vi "combined.vi"() -> ()   [LabVIEW 2020]
uses:
  C:/Users/Public/Documents/Photometrics/PMQI-LabViewSamples/Examples/2018/Dependencies/PVCamNET.dll
  Dependencies/PVCamNET.dll
panel:
  out "SavingPath":string
  out "Boolean 2":bool
  in  "seq_close":bool
  out "Capturing":bool
  in  "seq_save":bool
  in  "seq_start":bool
  in  "Path":path
  in  "FramesToCapture":u16
  in  "Full CCD Height":u16
  in  "Full CCD Width":u16
  in  "Full CCD":bool
  in  "Get ROI":bool
  in  "Height":u16
  in  "Y":u16
  in  "Width":u16
  in  "X":u16
  out "Trigger Mode":i32
  in  "Trigger In Behaviour":string(combo)
  out "Exp. out":i32
  in  "Trigger Out Behaviour":string(combo)
  out "Boolean":bool
  in  "Scan Direction Reset":bool
  out "Scan Line Time":dbl format="%#_14g"
  in  "Scan Width":dbl
  in  "Scan Line Delay":dbl
  in  "Scan Direction":string(combo)
  in  "Scan Mode":string(combo)
  in  "Exposure Time":dbl
  in  "Live":bool
  in  "Camera Status":bool
  in  "Uninit":bool
  in  "Live stop":bool
  in  "Live start":bool
  in  "Open":bool
  # "Description:\nThis code lets the user use programmable scan\n mode for live imaging.\n\nSteps to run:\n1. Click \"Run\"\n2. Click \"Open\"\n3. Enter Exposure Time\n4. Select Scan Mode. \n5. Set Scan Line Delay or Scan Width\n6. Select Scan Direction\n7. Click \"Live start\"\n8. Click \"Live stop\"\n9. Right click on CamWindow and add a ROI.\n10. Click \"Get ROI\"\n11. Click \"Live start\"\n12. Click \"Live stop\"\n13. Right click on CamWindow and delete a ROI.\n14. Click \"Close\""
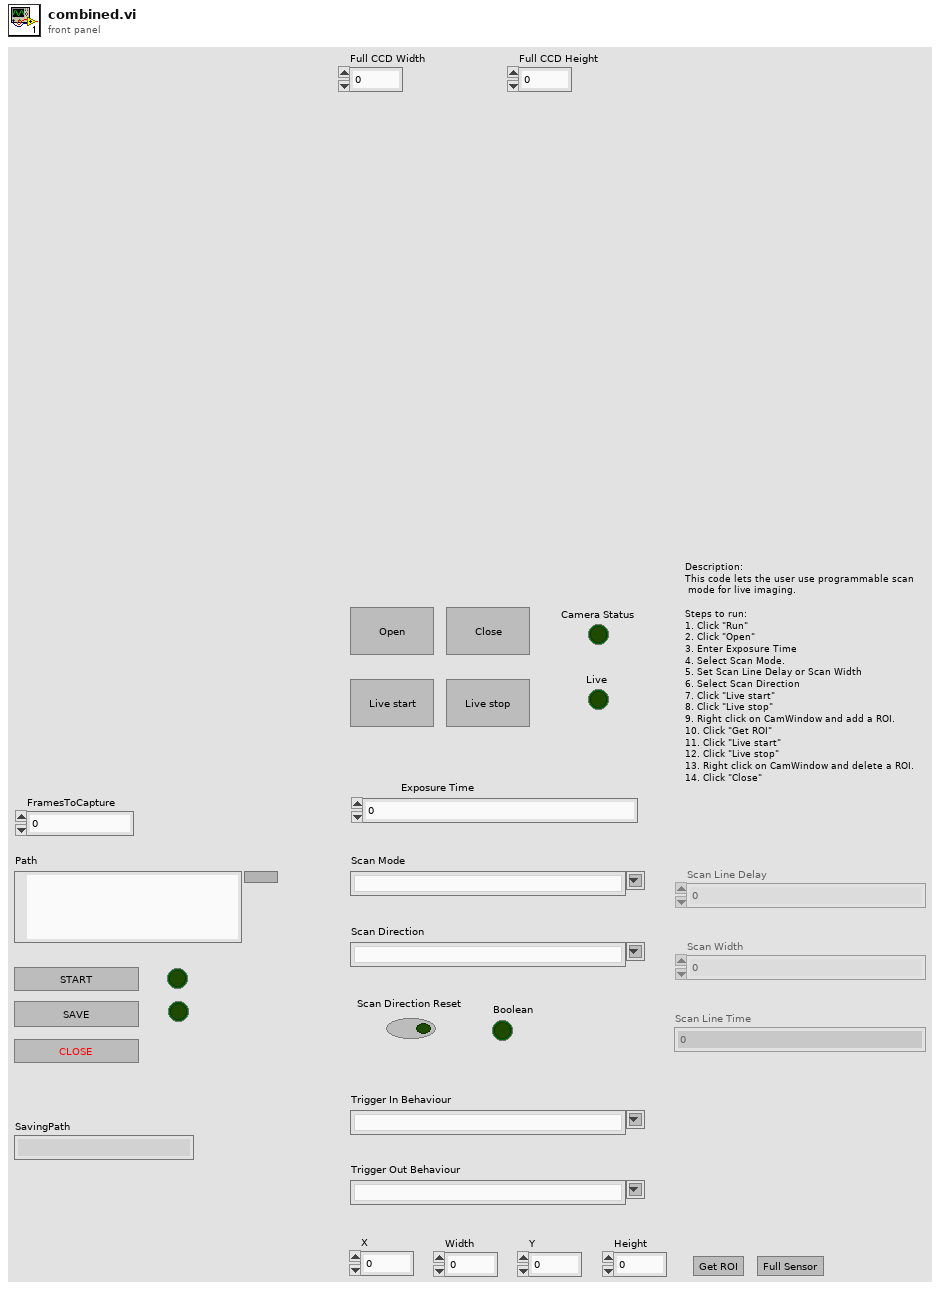
[diagram p1: front panel]
types:
  T1 = enum8{"Enabled", "Disabled", "Disabled and Grayed Out"}
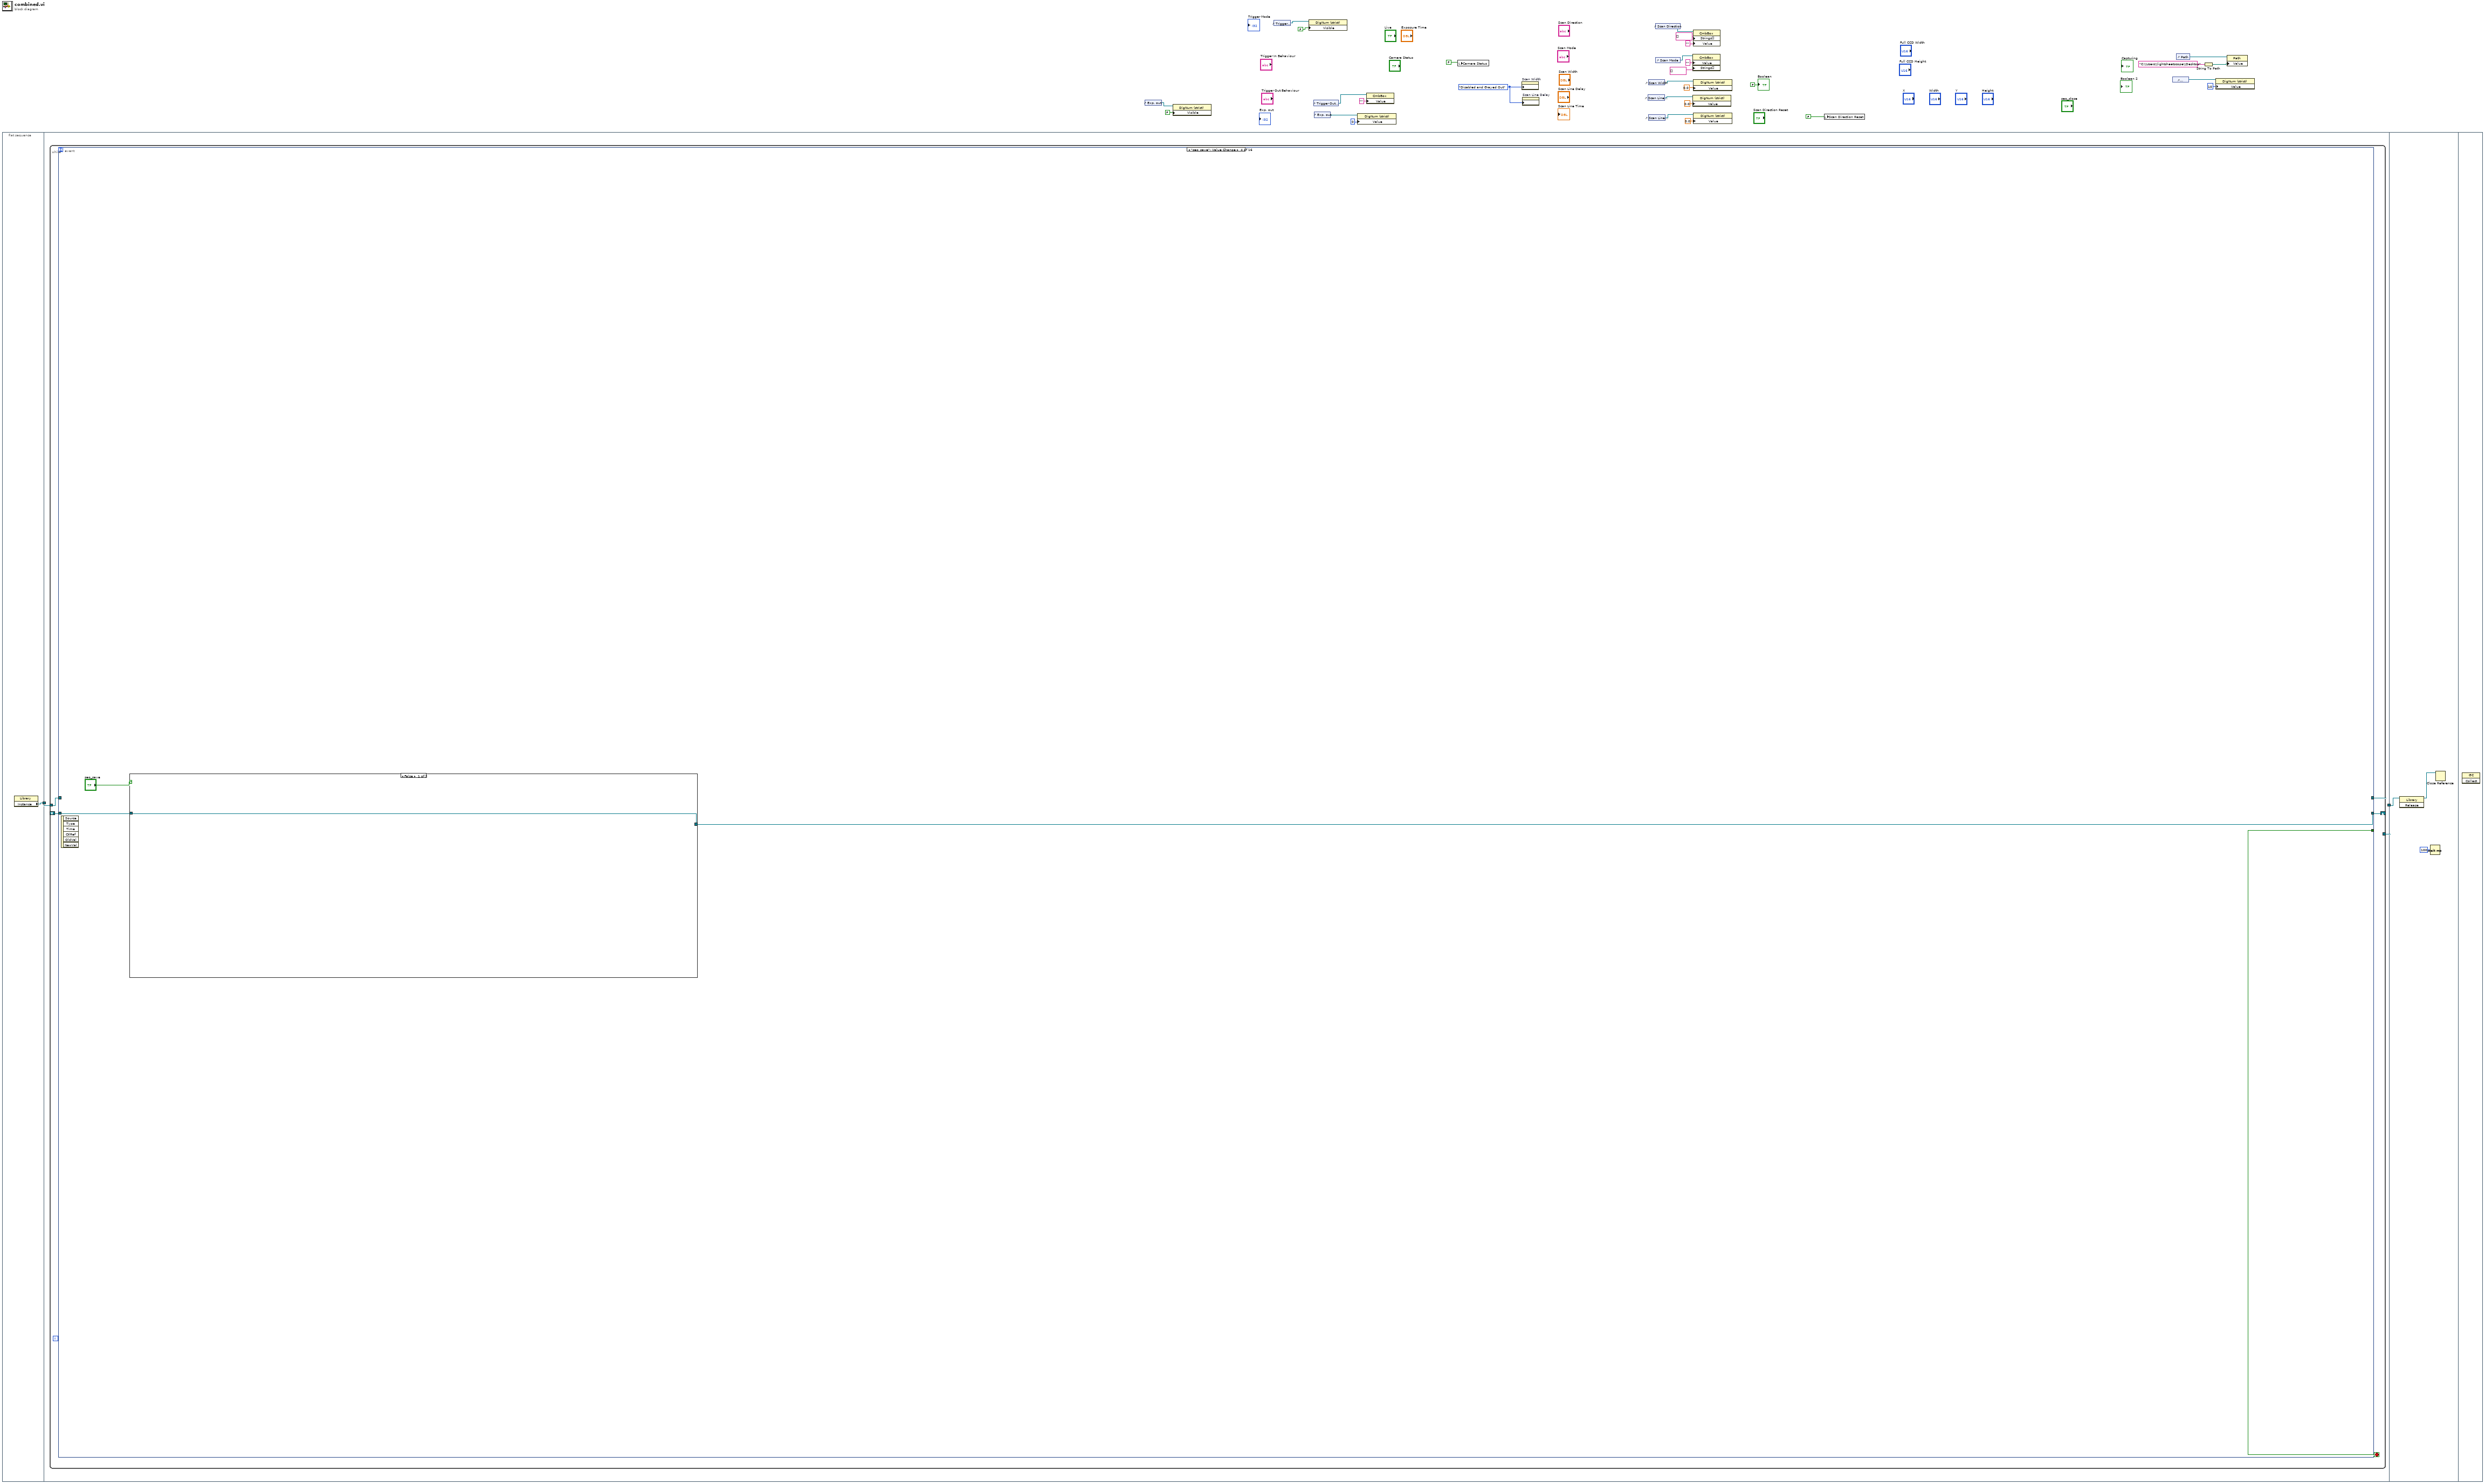
[diagram p0: block diagram]
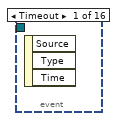
[diagram p2: hidden frame]
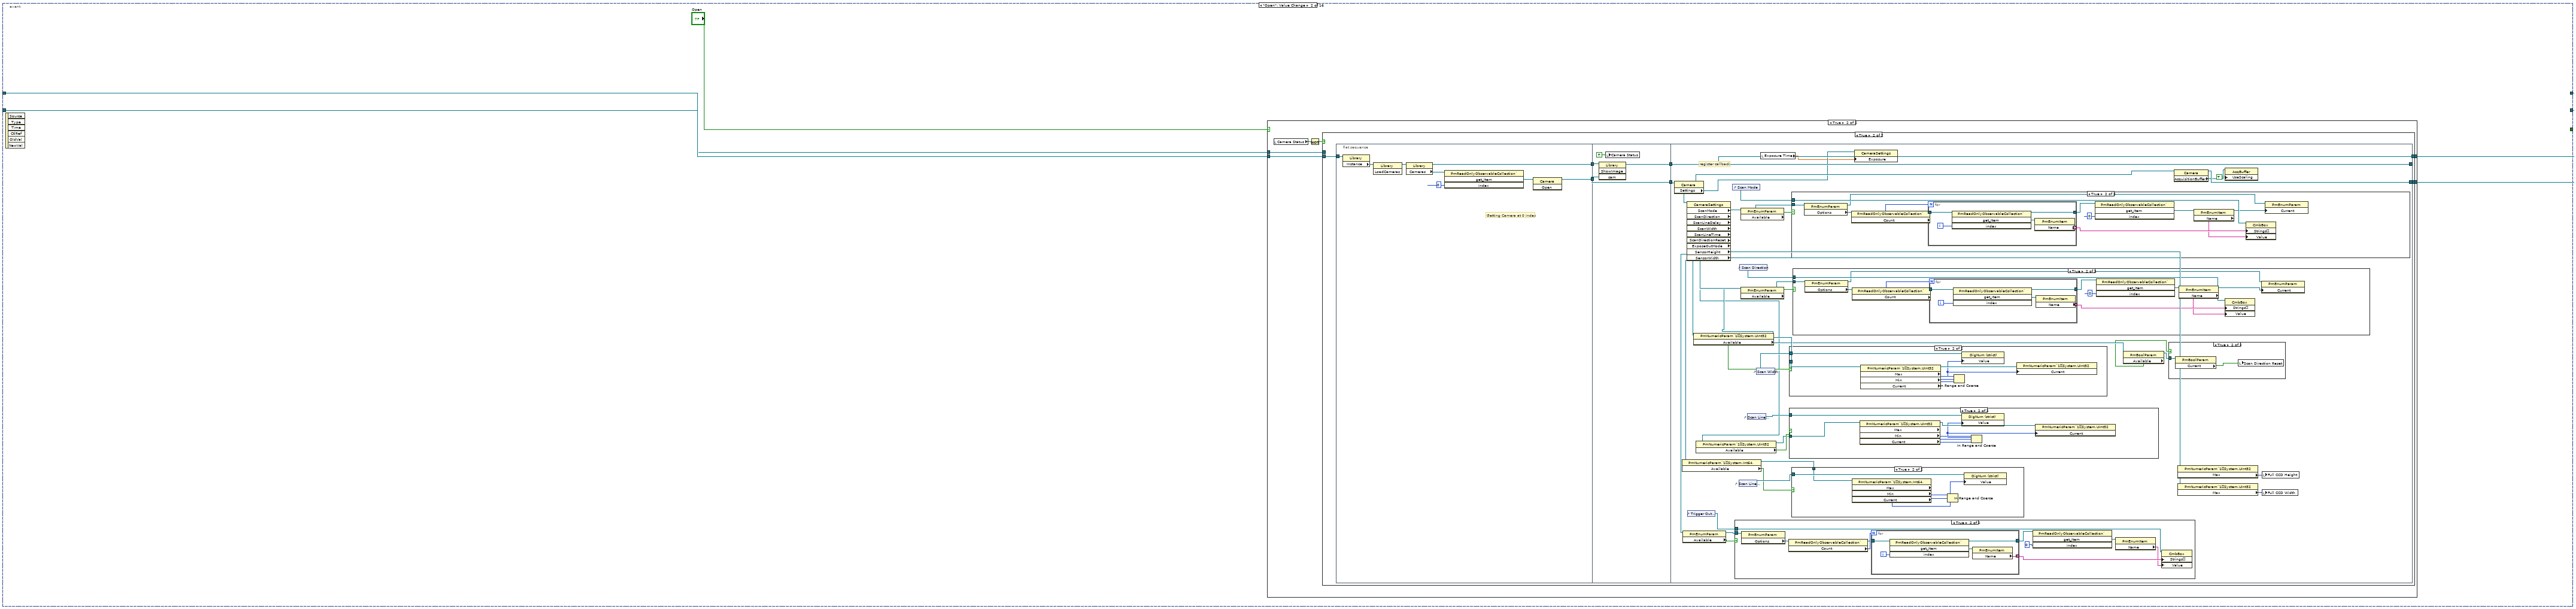
[diagram p3: hidden frame]
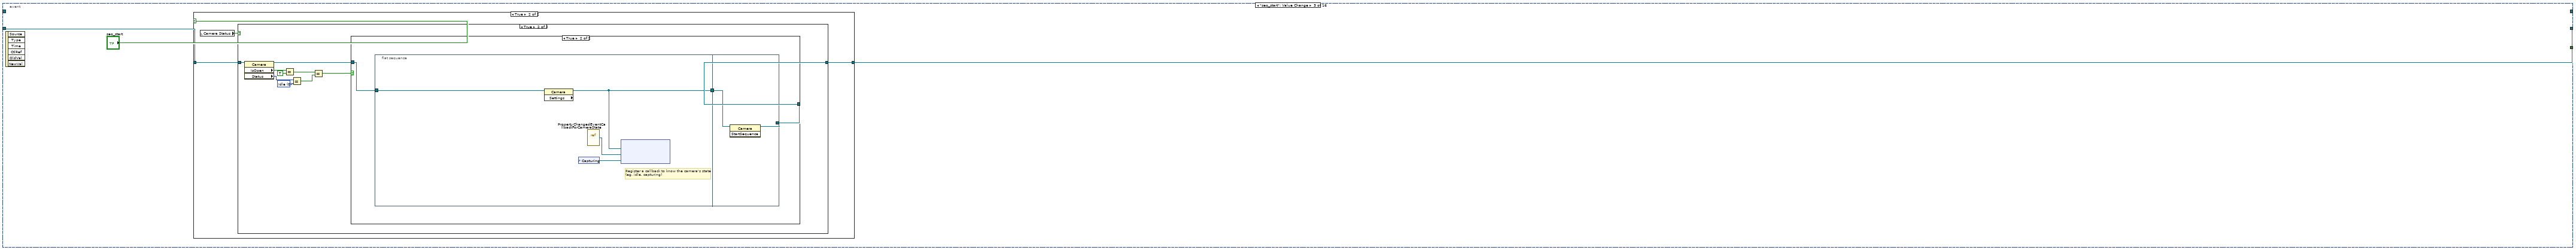
[diagram p13: hidden frame]
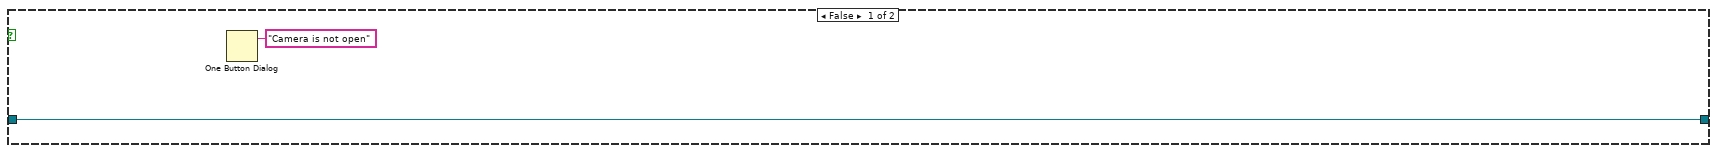
[diagram p15: hidden frame]
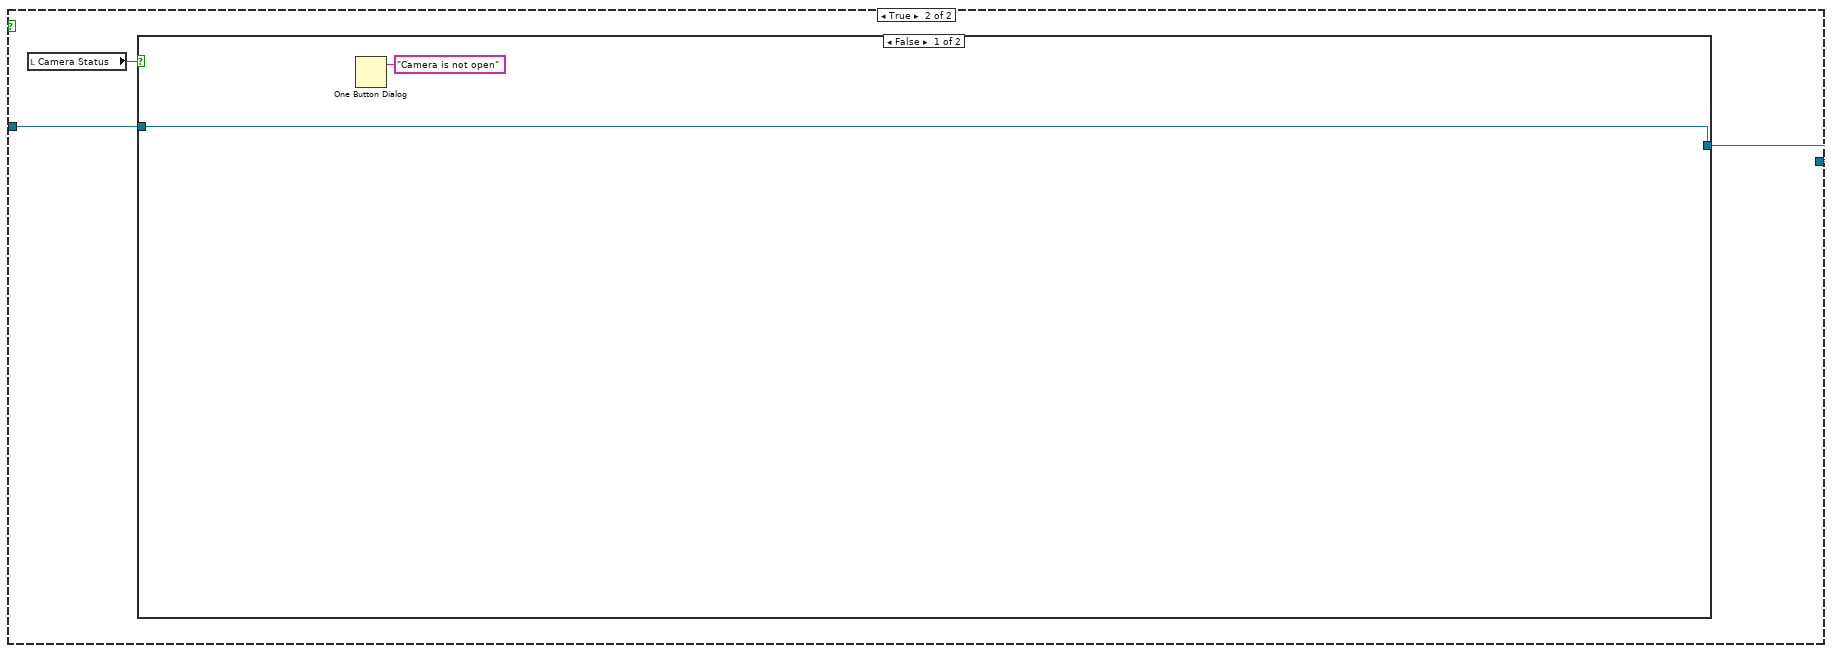
[diagram p17: hidden frame]
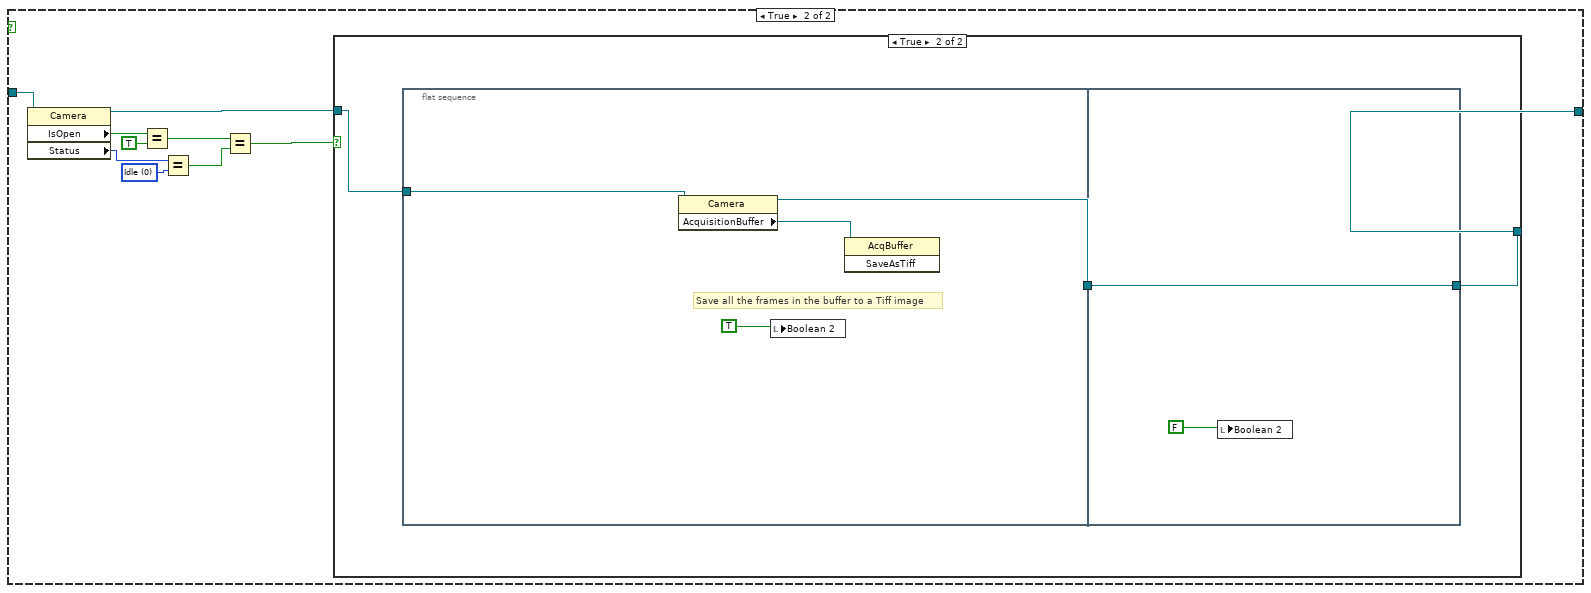
[diagram p18: hidden frame]
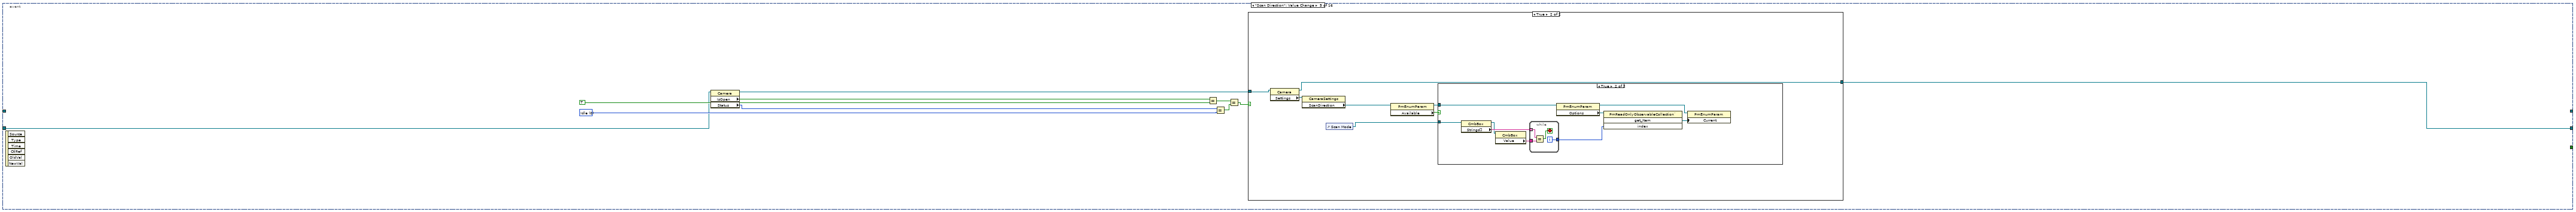
[diagram p20: hidden frame]
diagram:
  w16 = T1."Disabled and Grayed Out" ("Disabled")
  n1 = flat-sequence {
    tunnel: [w32] -> w31
    tunnel: w31 -> [w34]
    tunnel: [w33] -> w30
    tunnel: w30 -> [w855]
    frame #0 {
      n2 = property class="Library"() -> ("Instance"=w32:refnum<k24>)  [unwired: 2 in, 2 out]
    }
    frame #1 {
      n3 = while {
        tunnel: w34 -> [w39]
        shift-right: [w38] -> _
        shift-left: _ -> [w36]
        tunnel: [w37] -> w33
        stop <- w35 stop-if-true
        n4 = event shown="[3] \"seq_save\": Value Change" {
          selector: _ -> [_ _ _ _ _ _ _ _ _ _ _ _ _ _ _ _]
          dyn-events: _ -> [_ _ _ _ _ _ _ _ _ _ _ _ _ _ _ _]
          timeout: _ -> [_ _ _ _ _ _ _ _ _ _ _ _ _ _ _ _]
          tunnel: w39 -> [_ w44 _ _ _ _ _ _ w529 _ _ _ _ w772 _ w827]
          tunnel: [_ w43 w184 w215 w242 w274 w406 w470 w530 w597 w634 w707 w734 w773 w802 w828] -> w38
          tunnel: [_ w42 _ _ _ _ _ _ w529 _ _ _ _ w772 _ w827] -> w37
          tunnel: w36 -> [_ w41 w185 w214 w246 w275 w412 w472 w531 w598 w635 w708 w735 w774 w803 w829]
          tunnel: [_ _ _ _ _ _ _ _ _ _ _ _ _ _ _ w826] -> w35
          event Timeout {
            n5 = event-data() -> ()  [unwired: 1 in, 3 out]
          }
          event "Open": Value Change {
            n6 = event-data() -> ()  [unwired: 1 in, 6 out]
            n7 = case shown="True" "Open" {
              tunnel: w44 -> [w46 w52]
              tunnel: [w45 w51] -> w43
              tunnel: [w46 w50] -> w42
              tunnel: w41 -> [w45 w47]
              frame False {
              }
              frame True {
                n8 = local read "Camera Status"() -> (w49:bool)
                n9 = Not(x=w49) -> (.not. x?=w48:bool)
                n10 = case shown="True" w48 {
                  tunnel: w52 -> [w53 w59]
                  tunnel: [w54 w58] -> w51
                  tunnel: [w53 w57] -> w50
                  tunnel: w47 -> [w54 _]
                  frame False {
                  }
                  frame True {
                    n11 = flat-sequence {
                      tunnel: w59 -> [w64]
                      tunnel: [w66] -> w61
                      tunnel: [w65] -> w60
                      tunnel: w61 -> [w72]
                      tunnel: w60 -> [w73]
                      tunnel: [w73] -> w56
                      tunnel: [w71] -> w55
                      tunnel: [w112] -> w57
                      tunnel: [w92] -> w58
                      tunnel: w56 -> [w111]
                      tunnel: w55 -> [w112]
                      frame #0 {
                        # "Getting Camera at 0 index"
                        n12 = property class="Library"(reference=w64) -> ("Instance"=w63:refnum<k24>)  [unwired: 1 in, 2 out]
                        n13 = invoke class="Library" method="LoadCameras"(reference=w63) -> (reference out=w62:refnum<k24>)  [unwired: 2 in, 2 out]
                        n14 = property class="Library"(reference=w62) -> (reference out=w66:refnum<k24>, "Cameras"=w69:refnum<k24>)  [unwired: 1 in, 1 out]
                        n15 = invoke class="PmReadOnlyObservableCollection`" method="get_Item"(reference=w69, "index"=0) -> ("get_Item"=w67:refnum<k24>)  [unwired: 2 in, 3 out]
                        n16 = invoke class="Camera" method="Open"(reference=w67) -> (reference out=w65:refnum<k24>)  [unwired: 2 in, 2 out]
                      }
                      frame #1 {
                        n17 = invoke class="Library" method="ShowImage"(reference=w72, "cam"=w73) -> (reference out=w71:refnum<k24>)  [unwired: 2 in, 3 out]
                        n18 = local write "Camera Status"(TRUE ("Camera Status")) -> ()
                      }
                      frame #2 {
                        # "register callback"
                        n19 = property class="Camera"(reference=w111) -> (reference out=w93:refnum<k24>, "Settings"=w82:refnum<k24>)  [unwired: 1 in, 1 out]
                        n20 = property class="CameraSettings"(reference=w82) -> ("ScanMode"=w110:refnum<k24>, "ScanDirection"=w106:refnum<k24>, "ScanLineDelay"=w101:refnum<k24>, "ScanWidth"=w88:refnum<k24>, "ScanLineTime"=w80:refnum<k24>, "ScanDirectionReset"=w96:refnum<k24>, "ExposeOutMode"=w84:refnum<k24>, "SensorHeight"=w75:refnum<k24>, "SensorWidth"=w74:refnum<k24>)  [unwired: 1 in, 2 out]
                        n21 = property class="PmNumericParam`1[[System.Int64,"(reference=w80) -> (reference out=w78:refnum<k24>, "Available"=w79:bool)  [unwired: 1 in, 1 out]
                        n22 = property class="PmEnumParam"(reference=w84) -> (reference out=w85:refnum<k24>, "Available"=w86:bool)  [unwired: 1 in, 1 out]
                        n23 = control-ref of="Trigger Out Behaviour"() -> (w83:refnum<vi>)
                        n24 = property class="PmNumericParam`1[[System.UInt32"(reference=w101) -> (reference out=w99:refnum<k24>, "Available"=w100:bool)  [unwired: 1 in, 1 out]
                        n25 = property class="PmNumericParam`1[[System.UInt32"(reference=w88) -> (reference out=w87:refnum<k24>, "Available"=w89:bool)  [unwired: 1 in, 1 out]
                        n26 = control-ref of="Scan Mode"() -> (w107:refnum<vi>)
                        n27 = case shown="True" w86 {
                          tunnel: w85 -> [_ w122]
                          tunnel: w83 -> [_ w113]
                          frame False {
                          }
                          frame True {
                            n28 = property class="PmEnumParam"(reference=w122) -> ("Options"=w121:refnum<k24>)  [unwired: 1 in, 2 out]
                            n29 = property class="PmReadOnlyObservableCollection`"(reference=w121) -> (reference out=w119:refnum<k24>, "Count"=w120:i32)  [unwired: 1 in, 1 out]
                            n30 = for {
                              N: w120 -> [_]
                              tunnel: w119 -> [w127]
                              tunnel: [w124] -> w116
                              tunnel: [w123] -> w115 mode=indexing
                              i -> [w126]
                              n31 = invoke class="PmReadOnlyObservableCollection`" method="get_Item"(reference=w127, "index"=w126) -> (reference out=w124:refnum<k24>, "get_Item"=w125:refnum<k24>)  [unwired: 2 in, 2 out]
                              n32 = property class="PmEnumItem"(reference=w125) -> ("Name"=w123:string)  [unwired: 1 in, 2 out]
                            }
                            n33 = invoke class="PmReadOnlyObservableCollection`" method="get_Item"(reference=w116, "index"=0) -> ("get_Item"=w117:refnum<k24>)  [unwired: 2 in, 3 out]
                            n34 = property class="PmEnumItem"(reference=w117) -> ("Name"=w114:string)  [unwired: 1 in, 2 out]
                            n35 = property class="CmbBox"(reference=w113, "Strings[]"=w115, "Value"=w114) -> ()  [unwired: 1 in, 2 out]
                          }
                        }
                        n36 = control-ref of="Scan Line Time"() -> (w97:refnum<vi>)
                        n37 = control-ref of="Scan Direction"() -> (w103:refnum<vi>)
                        n38 = property class="PmEnumParam"(reference=w110) -> (reference out=w108:refnum<k24>, "Available"=w109:bool)  [unwired: 1 in, 1 out]
                        n39 = property class="PmEnumParam"(reference=w106) -> (reference out=w104:refnum<k24>, "Available"=w105:bool)  [unwired: 1 in, 1 out]
                        n40 = control-ref of="Scan Line Delay"() -> (w98:refnum<vi>)
                        n41 = control-ref of="Scan Width"() -> (w102:refnum<vi>)
                        n42 = local read "Exposure Time"() -> (w81:dbl)
                        n43 = case shown="True" w89 {
                          tunnel: w98 -> [_ w139]
                          tunnel: w87 -> [_ w138]
                          frame False {
                          }
                          frame True {
                            n44 = property class="PmNumericParam`1[[System.UInt32"(reference=w138) -> (reference out=w137:refnum<k24>, "Max"=w140:u32, "Min"=w141:u32, "Current"=w142:u32)  [unwired: 1 in, 1 out]
                            n45 = In Range and Coerce(upper limit=w140, x=w142, lower limit=w141) -> (coerced(x)=w136:u32)  [unwired: 1 out]
                            n46 = property class="DigNum (strict)"(reference=w139, "Value"=w136) -> ()  [unwired: 1 in, 2 out]
                            n47 = property class="PmNumericParam`1[[System.UInt32"(reference=w137, "Current"=w136) -> ()  [unwired: 1 in, 2 out]
                          }
                        }
                        n48 = case shown="True" w100 {
                          tunnel: w102 -> [_ w146]
                          tunnel: w99 -> [_ w145]
                          frame False {
                          }
                          frame True {
                            n49 = property class="PmNumericParam`1[[System.UInt32"(reference=w145) -> (reference out=w144:refnum<k24>, "Max"=w147:u32, "Min"=w148:u32, "Current"=w149:u32)  [unwired: 1 in, 1 out]
                            n50 = In Range and Coerce(upper limit=w147, x=w149, lower limit=w148) -> (coerced(x)=w143:u32)  [unwired: 1 out]
                            n51 = property class="DigNum (strict)"(reference=w146, "Value"=w143) -> ()  [unwired: 1 in, 2 out]
                            n52 = property class="PmNumericParam`1[[System.UInt32"(reference=w144, "Current"=w143) -> ()  [unwired: 1 in, 2 out]
                          }
                        }
                        n53 = case shown="True" w79 {
                          tunnel: w97 -> [_ w131]
                          tunnel: w78 -> [_ w130]
                          frame False {
                          }
                          frame True {
                            n54 = property class="PmNumericParam`1[[System.Int64,"(reference=w130) -> ("Max"=w132:i64, "Min"=w133:i64, "Current"=w134:i64)  [unwired: 1 in, 2 out]
                            n55 = In Range and Coerce(upper limit=w132, x=w134, lower limit=w133) -> (coerced(x)=w135:i64)  [unwired: 1 out]
                            n56 = property class="DigNum (strict)"(reference=w131, "Value"=w135) -> ()  [unwired: 1 in, 2 out]
                          }
                        }
                        n57 = case shown="True" w109 {
                          tunnel: w108 -> [_ w178]
                          tunnel: w107 -> [_ w170]
                          frame False {
                          }
                          frame True {
                            n58 = property class="PmEnumParam"(reference=w178) -> (reference out=w169:refnum<k24>, "Options"=w177:refnum<k24>)  [unwired: 1 in, 1 out]
                            n59 = property class="PmReadOnlyObservableCollection`"(reference=w177) -> (reference out=w175:refnum<k24>, "Count"=w176:i32)  [unwired: 1 in, 1 out]
                            n60 = for {
                              N: w176 -> [_]
                              tunnel: w175 -> [w183]
                              tunnel: [w180] -> w173
                              tunnel: [w179] -> w172 mode=indexing
                              i -> [w182]
                              n61 = invoke class="PmReadOnlyObservableCollection`" method="get_Item"(reference=w183, "index"=w182) -> (reference out=w180:refnum<k24>, "get_Item"=w181:refnum<k24>)  [unwired: 2 in, 2 out]
                              n62 = property class="PmEnumItem"(reference=w181) -> ("Name"=w179:string)  [unwired: 1 in, 2 out]
                            }
                            n63 = invoke class="PmReadOnlyObservableCollection`" method="get_Item"(reference=w173, "index"=0) -> ("get_Item"=w168:refnum<k24>)  [unwired: 2 in, 3 out]
                            n64 = property class="PmEnumItem"(reference=w168) -> (reference out=w167:refnum<k24>, "Name"=w171:string)  [unwired: 1 in, 1 out]
                            n65 = property class="CmbBox"(reference=w170, "Strings[]"=w172, "Value"=w171) -> ()  [unwired: 1 in, 2 out]
                            n66 = property class="PmEnumParam"(reference=w169, "Current"=w167) -> ()  [unwired: 1 in, 2 out]
                          }
                        }
                        n67 = case shown="True" w105 {
                          tunnel: w104 -> [_ w161]
                          tunnel: w103 -> [_ w152]
                          frame False {
                          }
                          frame True {
                            n68 = property class="PmEnumParam"(reference=w161) -> (reference out=w151:refnum<k24>, "Options"=w160:refnum<k24>)  [unwired: 1 in, 1 out]
                            n69 = property class="PmReadOnlyObservableCollection`"(reference=w160) -> (reference out=w158:refnum<k24>, "Count"=w159:i32)  [unwired: 1 in, 1 out]
                            n70 = for {
                              N: w159 -> [_]
                              tunnel: w158 -> [w166]
                              tunnel: [w163] -> w155
                              tunnel: [w162] -> w154 mode=indexing
                              i -> [w165]
                              n71 = invoke class="PmReadOnlyObservableCollection`" method="get_Item"(reference=w166, "index"=w165) -> (reference out=w163:refnum<k24>, "get_Item"=w164:refnum<k24>)  [unwired: 2 in, 2 out]
                              n72 = property class="PmEnumItem"(reference=w164) -> ("Name"=w162:string)  [unwired: 1 in, 2 out]
                            }
                            n73 = invoke class="PmReadOnlyObservableCollection`" method="get_Item"(reference=w155, "index"=0) -> ("get_Item"=w156:refnum<k24>)  [unwired: 2 in, 3 out]
                            n74 = property class="PmEnumItem"(reference=w156) -> (reference out=w150:refnum<k24>, "Name"=w153:string)  [unwired: 1 in, 1 out]
                            n75 = property class="CmbBox"(reference=w152, "Strings[]"=w154, "Value"=w153) -> ()  [unwired: 1 in, 2 out]
                            n76 = property class="PmEnumParam"(reference=w151, "Current"=w150) -> ()  [unwired: 1 in, 2 out]
                          }
                        }
                        n77 = property class="CameraSettings"(reference=w82, "Exposure"=w81) -> ()  [unwired: 1 in, 2 out]
                        n78 = property class="PmBoolParam"(reference=w96) -> (reference out=w94:refnum<k24>, "Available"=w95:bool)  [unwired: 1 in, 1 out]
                        n79 = case shown="True" w95 {
                          tunnel: w94 -> [_ w129]
                          frame False {
                          }
                          frame True {
                            n80 = property class="PmBoolParam"(reference=w129) -> ("Current"=w128:bool)  [unwired: 1 in, 2 out]
                            n81 = local write "Scan Direction Reset"(w128) -> ()
                          }
                        }
                        n82 = property class="Camera"(reference=w93) -> (reference out=w92:refnum<k24>, "AcquisitionBuffer"=w91:refnum<k24>)  [unwired: 1 in, 1 out]
                        n83 = property class="PmNumericParam`1[[System.UInt32"(reference=w75) -> ("Max"=w77:u32)  [unwired: 1 in, 2 out]
                        n84 = property class="PmNumericParam`1[[System.UInt32"(reference=w74) -> ("Max"=w76:u32)  [unwired: 1 in, 2 out]
                        n85 = property class="AcqBuffer"(reference=w91, "UseScaling"=TRUE) -> ()  [unwired: 1 in, 2 out]
                        n86 = local write "Full CCD Height"(w77) -> ()
                        n87 = local write "Full CCD Width"(w76) -> ()
                      }
                    }
                  }
                }
              }
            }
          }
          event "seq_start": Value Change {
            n88 = event-data() -> ()  [unwired: 1 in, 6 out]
            n89 = case shown="True" "seq_start" {
              tunnel: w185 -> [w187 w190]
              tunnel: [w187 w188] -> w184
              frame False {
              }
              frame True {
                n90 = local read "Camera Status"() -> (w189:bool)
                n91 = case shown="True" w189 {
                  tunnel: w190 -> [w191 w196]
                  tunnel: [w191 w193] -> w188
                  frame False {
                    n92 = One Button Dialog(message="Camera is not open") -> ()  [unwired: 1 in, 1 out]
                  }
                  frame True {
                    w201 = 0 items=["Idle", "Capturing"] ("Status")
                    n93 = property class="Camera"(reference=w196) -> (reference out=w195:refnum<k24>, "IsOpen"=w200:bool, "Status"=w202:i32)  [unwired: 1 in, 1 out]
                    n94 = Equal?(x=w200, y=TRUE) -> (x = y?=w198:bool)
                    n95 = Equal?(x=w202, y=w201) -> (x = y?=w197:bool)
                    n96 = Equal?(x=w198, y=w197) -> (x = y?=w194:bool)
                    n97 = case shown="True" w194 {
                      tunnel: w195 -> [w203 w206]
                      tunnel: [w203 w204] -> w193
                      frame False {
                      }
                      frame True {
                        n98 = flat-sequence {
                          tunnel: w206 -> [w208]
                          tunnel: [w207] -> w205
                          tunnel: [w212] -> w204
                          tunnel: w205 -> [w211]
                          frame #0 {
                            # "Register a callback to know the camera's state \n(eg. idle, capturing)"
                            n99 = property class="Camera" props=["Settings"](reference=w208) -> (reference out=w207:refnum<k24>)  [unwired: 1 in, 2 out]
                            n100 = control-ref of="Capturing"() -> (w209:refnum<vi>)
                            n101 = vi-ref "PropertyChangedEventCallbackForCameraState.vi"() -> ("vi reference"=w210:refnum<vi>)
                            n102 = node(w207, w210, w209) -> ()  [unwired: 2 in, 2 out]
                          }
                          frame #1 {
                            n103 = invoke class="Camera" method="StartSequence"(reference=w211) -> (reference out=w212:refnum<k24>)  [unwired: 2 in, 2 out]
                          }
                        }
                      }
                    }
                  }
                }
              }
            }
          }
          event "seq_save": Value Change {
            n104 = event-data() -> ()  [unwired: 1 in, 6 out]
            n105 = case shown="False" "seq_save" {
              tunnel: [w216 w218] -> w215
              tunnel: w214 -> [w216 w217]
              frame False {
              }
              frame True {
                n106 = local read "Camera Status"() -> (w219:bool)
                n107 = case shown="False" w219 {
                  tunnel: [w220 w223] -> w218
                  tunnel: w217 -> [w220 w222]
                  frame False {
                    n108 = One Button Dialog(message="Camera is not open") -> ()  [unwired: 1 in, 1 out]
                  }
                  frame True {
                    w230 = 0 items=["Idle", "Capturing"] ("Status")
                    n109 = property class="Camera"(reference=w222) -> (reference out=w225:refnum<k24>, "IsOpen"=w229:bool, "Status"=w231:i32)  [unwired: 1 in, 1 out]
                    n110 = Equal?(x=w229, y=TRUE) -> (x = y?=w227:bool)
                    n111 = Equal?(x=w231, y=w230) -> (x = y?=w226:bool)
                    n112 = Equal?(x=w227, y=w226) -> (x = y?=w224:bool)
                    n113 = case shown="True" w224 {
                      tunnel: w225 -> [w232 w235]
                      tunnel: [w232 w234] -> w223
                      frame False {
                      }
                      frame True {
                        n114 = flat-sequence {
                          tunnel: [w237] -> w233
                          tunnel: w235 -> [w236]
                          tunnel: [w240] -> w234
                          tunnel: w233 -> [w240]
                          frame #0 {
                            # "Save all the frames in the buffer to a Tiff image"
                            n115 = property class="Camera"(reference=w236) -> (reference out=w237:refnum<k24>, "AcquisitionBuffer"=w239:refnum<k24>)  [unwired: 1 in, 1 out]
                            n116 = local write "Boolean 2"(TRUE ("Camera Status")) -> ()
                            n117 = invoke class="AcqBuffer" method="SaveAsTiff"(reference=w239) -> ()  [unwired: 2 in, 3 out]
                          }
                          frame #1 {
                            n118 = local write "Boolean 2"(FALSE ("Camera Status")) -> ()
                          }
                        }
                      }
                    }
                  }
                }
              }
            }
          }
          event "Scan Direction": Value Change {
            w250 = 0 items=["Idle", "Capturing"] ("Status")
            n119 = event-data() -> ()  [unwired: 1 in, 6 out]
            n120 = property class="Camera"(reference=w246) -> (reference out=w243:refnum<k24>, "IsOpen"=w249:bool, "Status"=w251:i32)  [unwired: 1 in, 1 out]
            n121 = Equal?(x=w249, y=TRUE) -> (x = y?=w245:bool)
            n122 = Equal?(x=w251, y=w250) -> (x = y?=w247:bool)
            n123 = Equal?(x=w245, y=w247) -> (x = y?=w244:bool)
            n124 = case shown="True" w244 {
              tunnel: w243 -> [w252 w256]
              tunnel: [w252 w253] -> w242
              frame False {
              }
              frame True {
                n125 = property class="Camera"(reference=w256) -> (reference out=w253:refnum<k24>, "Settings"=w257:refnum<k24>)  [unwired: 1 in, 1 out]
                n126 = property class="CameraSettings"(reference=w257) -> ("ScanDirection"=w255:refnum<k24>)  [unwired: 1 in, 2 out]
                n127 = control-ref of="Scan Mode"() -> (w254:refnum<vi>)
                n128 = property class="PmEnumParam"(reference=w255) -> (reference out=w258:refnum<k24>, "Available"=w259:bool)  [unwired: 1 in, 1 out]
                n129 = case shown="True" w259 {
                  tunnel: w258 -> [_ w267]
                  tunnel: w254 -> [_ w260]
                  frame False {
                  }
                  frame True {
                    n130 = property class="CmbBox"(reference=w260) -> (reference out=w262:refnum<vi>, "Strings[]"=w268:string[])  [unwired: 1 in, 1 out]
                    n131 = property class="CmbBox"(reference=w262) -> ("Value"=w261:string)  [unwired: 1 in, 2 out]
                    n132 = while {
                      tunnel: w268 -> [w272] mode=indexing
                      tunnel: [w270] -> w265
                      tunnel: w261 -> [w269]
                      i -> [w270]
                      stop <- w271 stop-if-true
                      n133 = Equal?(x=w272, y=w269) -> (x = y?=w271:bool)
                    }
                    n134 = property class="PmEnumParam"(reference=w267) -> (reference out=w264:refnum<k24>, "Options"=w266:refnum<k24>)  [unwired: 1 in, 1 out]
                    n135 = invoke class="PmReadOnlyObservableCollection`" method="get_Item"(reference=w266, "index"=w265) -> ("get_Item"=w263:refnum<k24>)  [unwired: 2 in, 3 out]
                    n136 = property class="PmEnumParam"(reference=w264, "Current"=w263) -> ()  [unwired: 1 in, 2 out]
                  }
                }
              }
            }
          }
          event "Scan Mode", "Scan Direction Reset": Value Change {
            n137 = event-data() -> ()  [unwired: 1 in, 6 out]
            n138 = local read "Camera Status"() -> (w273:bool)
            n139 = case shown="True" w273 {
              tunnel: w275 -> [w276 w281]
              tunnel: [w276 w279] -> w274
              frame False {
                n140 = One Button Dialog(message="Camera is not open") -> ()  [unwired: 1 in, 1 out]
              }
              frame True {
                w286 = 0 items=["Idle", "Capturing"] ("Status")
                n141 = property class="Camera"(reference=w281) -> (reference out=w280:refnum<k24>, "IsOpen"=w285:bool, "Status"=w287:i32)  [unwired: 1 in, 1 out]
                n142 = Equal?(x=w285, y=TRUE) -> (x = y?=w283:bool)
                n143 = Equal?(x=w287, y=w286) -> (x = y?=w282:bool)
                n144 = Equal?(x=w283, y=w282) -> (x = y?=w278:bool)
                n145 = case shown="True" w278 {
                  tunnel: w280 -> [w288 w327]
                  tunnel: [w288 w322] -> w279
                  frame False {
                  }
                  frame True {
                    # "For Scan mode type if Auto is chosen then Scan Width and Scan Line Delay are not configurable.\nIf Line Delay is chosen then Scan Line is configurable, but Scan Width is not configurable.\nSimilarly if Scan Delay is chosen then Scan Line Delay is configurable, but Scan Width is not configurable."
                    n146 = property class="Camera"(reference=w327) -> (reference out=w322:refnum<k24>, "Settings"=w326:refnum<k24>)  [unwired: 1 in, 1 out]
                    n147 = property class="CameraSettings"(reference=w326) -> (error out=w319:errorcluster, "ScanMode"=w325:refnum<k24>, "ScanDirection"=w321:refnum<k24>, "ScanWidth"=w317:refnum<k24>, "ScanLineDelay"=w316:refnum<k24>, "ScanLineTime"=w305:refnum<k24>, "ScanDirectionReset"=w294:refnum<k24>)  [unwired: 1 in, 1 out]
                    n148 = control-ref of="Scan Line Delay"() -> (w296:refnum<vi>)
                    n149 = control-ref of="Scan Line Time"() -> (w299:refnum<vi>)
                    n150 = control-ref of="Scan Width"() -> (w312:refnum<vi>)
                    n151 = property class="PmEnumParam"(reference=w325, error in=w319) -> (reference out=w323:refnum<k24>, error out=w320:errorcluster, "Available"=w324:bool)
                    n152 = control-ref of="Scan Mode"() -> (w318:refnum<vi>)
                    n153 = control-ref of="Scan Direction"() -> (w315:refnum<vi>)
                    n154 = case shown="True" w324 {
                      tunnel: w323 -> [_ w400]
                      tunnel: w318 -> [_ w395]
                      tunnel: w320 -> [w388 w394]
                      tunnel: [w388 w389] -> w304
                      frame False {
                      }
                      frame True {
                        n155 = property class="CmbBox"(reference=w395) -> (reference out=w396:refnum<vi>, "Strings[]"=w401:string[])  [unwired: 1 in, 1 out]
                        n156 = property class="CmbBox"(reference=w396) -> ("Value"=w391:string)  [unwired: 1 in, 2 out]
                        n157 = while {
                          tunnel: w401 -> [w405] mode=indexing
                          tunnel: [w403] -> w398
                          tunnel: w391 -> [w402]
                          i -> [w403]
                          stop <- w404 stop-if-true
                          n158 = Equal?(x=w405, y=w402) -> (x = y?=w404:bool)
                        }
                        n159 = property class="PmEnumParam"(reference=w400, error in=w394) -> (reference out=w397:refnum<k24>, error out=w393:errorcluster, "Options"=w399:refnum<k24>)
                        n160 = invoke class="PmReadOnlyObservableCollection`" method="get_Item"(reference=w399, error in=w393, "index"=w398) -> (error out=w392:errorcluster, "get_Item"=w390:refnum<k24>)  [unwired: 1 in, 2 out]
                        n161 = property class="PmEnumParam" props=["Current", "IsReadOnly"](reference=w397, error in=w392, "Current"=w390) -> (error out=w389:errorcluster)  [unwired: 2 out]
                      }
                    }
                    n162 = property class="PmEnumParam"(reference=w321, error in=w304) -> (reference out=w313:refnum<k24>, error out=w307:errorcluster, "Available"=w314:bool)
                    n163 = case shown="True" w314 {
                      tunnel: w313 -> [_ w382]
                      tunnel: w315 -> [_ w374]
                      tunnel: w307 -> [w366 w373]
                      tunnel: [w366 w367] -> w306
                      frame False {
                      }
                      frame True {
                        n164 = property class="PmEnumParam"(reference=w382, error in=w373) -> (reference out=w368:refnum<k24>, error out=w372:errorcluster, "Options"=w381:refnum<k24>)
                        n165 = property class="PmReadOnlyObservableCollection`"(reference=w381) -> (reference out=w379:refnum<k24>, "Count"=w380:i32)  [unwired: 1 in, 1 out]
                        n166 = for {
                          N: w380 -> [_]
                          tunnel: w379 -> [w387]
                          tunnel: [w384] -> w377
                          tunnel: [w383] -> w376 mode=indexing
                          i -> [w386]
                          n167 = invoke class="PmReadOnlyObservableCollection`" method="get_Item"(reference=w387, "index"=w386) -> (reference out=w384:refnum<k24>, "get_Item"=w385:refnum<k24>)  [unwired: 2 in, 2 out]
                          n168 = property class="PmEnumItem"(reference=w385) -> ("Name"=w383:string)  [unwired: 1 in, 2 out]
                        }
                        n169 = invoke class="PmReadOnlyObservableCollection`" method="get_Item"(reference=w377, error in=w372, "index"=0) -> (error out=w371:errorcluster, "get_Item"=w369:refnum<k24>)  [unwired: 1 in, 2 out]
                        n170 = property class="PmEnumItem"(reference=w369, error in=w371) -> (error out=w370:errorcluster, "Name"=w375:string)  [unwired: 1 out]
                        n171 = property class="CmbBox"(reference=w374, error in=w370, "Strings[]"=w376, "Value"=w375) -> (error out=w367:errorcluster)  [unwired: 1 out]
                        n172 = property class="PmEnumParam"(reference=w368, "Current"=w369) -> ()  [unwired: 1 in, 2 out]
                      }
                    }
                    n173 = property class="PmNumericParam`1[[System.UInt32"(reference=w317, error in=w306) -> (reference out=w310:refnum<k24>, error out=w309:errorcluster, "Available"=w311:bool)
                    n174 = case shown="True" w311 {
                      tunnel: w312 -> [_ w362]
                      tunnel: w310 -> [_ w359]
                      tunnel: w309 -> [w356 w361]
                      tunnel: [w356 w360] -> w308
                      frame False {
                      }
                      frame True {
                        n175 = property class="PmNumericParam`1[[System.UInt32"(reference=w359) -> ("Current"=w363:u32, "IsReadOnly"=w358:bool)  [unwired: 1 in, 2 out]
                        n176 = case shown="False" w358 {
                          tunnel: [T1."Enabled" ("Disabled") T1."Disabled and Grayed Out" ("Disabled")] -> w357
                          frame False {
                          }
                          frame True {
                          }
                        }
                        n177 = property class="DigNum (strict)"(reference=w362, error in=w361, "Value"=w363, "DisabledEnum"=w357) -> (error out=w360:errorcluster)  [unwired: 1 out]
                      }
                    }
                    n178 = property class="PmNumericParam`1[[System.UInt32"(reference=w316, error in=w308) -> (reference out=w301:refnum<k24>, error out=w295:errorcluster, "Available"=w302:bool)
                    n179 = case shown="True" w302 {
                      tunnel: w296 -> [_ w352]
                      tunnel: w301 -> [_ w349]
                      tunnel: w295 -> [w346 w351]
                      tunnel: [w346 w350] -> w298
                      frame False {
                      }
                      frame True {
                        n180 = property class="PmNumericParam`1[[System.UInt32"(reference=w349) -> ("Current"=w353:u32, "IsReadOnly"=w348:bool)  [unwired: 1 in, 2 out]
                        n181 = case shown="False" w348 {
                          tunnel: [T1."Enabled" ("Disabled") T1."Disabled and Grayed Out" ("Disabled")] -> w347
                          frame False {
                          }
                          frame True {
                          }
                        }
                        n182 = property class="DigNum (strict)"(reference=w352, error in=w351, "Value"=w353, "DisabledEnum"=w347) -> (error out=w350:errorcluster)  [unwired: 1 out]
                      }
                    }
                    n183 = property class="PmNumericParam`1[[System.Int64,"(reference=w305, error in=w298) -> (reference out=w300:refnum<k24>, error out=w297:errorcluster, "Available"=w303:bool)
                    n184 = case shown="True" w303 {
                      tunnel: w299 -> [_ w342]
                      tunnel: w300 -> [_ w339]
                      tunnel: w297 -> [w336 w341]
                      tunnel: [w336 w340] -> w290
                      frame False {
                      }
                      frame True {
                        n185 = property class="PmNumericParam`1[[System.Int64,"(reference=w339) -> ("Current"=w343:i64, "IsReadOnly"=w338:bool)  [unwired: 1 in, 2 out]
                        n186 = case shown="False" w338 {
                          tunnel: [T1."Enabled" ("Disabled") T1."Disabled and Grayed Out" ("Disabled")] -> w337
                          frame False {
                          }
                          frame True {
                          }
                        }
                        n187 = property class="DigNum (strict)"(reference=w342, error in=w341, "Value"=w343, "DisabledEnum"=w337) -> (error out=w340:errorcluster)  [unwired: 1 out]
                      }
                    }
                    n188 = property class="PmBoolParam"(reference=w294, error in=w290) -> (reference out=w292:refnum<k24>, error out=w289:errorcluster, "Available"=w293:bool)
                    n189 = control-ref of="Scan Direction Reset"() -> (w291:refnum<vi>)
                    n190 = case shown="True" w293 {
                      tunnel: w292 -> [_ w333]
                      tunnel: w291 -> [_ w335]
                      tunnel: w289 -> [_ w330]
                      frame False {
                      }
                      frame True {
                        n191 = property class="Bool (strict)"(reference=w335, error in=w330) -> (error out=w329:errorcluster, "Value"=w334:bool)  [unwired: 1 out]
                        n192 = property class="PmBoolParam"(reference=w333, error in=w329, "Current"=w334) -> (reference out=w332:refnum<k24>, error out=w328:errorcluster)
                        n193 = property class="PmBoolParam"(reference=w332, error in=w328) -> ("Current"=w331:bool)  [unwired: 2 out]
                        n194 = local write "Boolean"(w331) -> ()
                      }
                    }
                  }
                }
              }
            }
          }
          event "Scan Line Delay": Value Change {
            w417 = 0 items=["Idle", "Capturing"] ("Status")
            n195 = event-data() -> ()  [unwired: 1 in, 6 out]
            n196 = property class="Camera"(reference=w412) -> (reference out=w411:refnum<k24>, "IsOpen"=w416:bool, "Status"=w418:i32)  [unwired: 1 in, 1 out]
            n197 = Equal?(x=w416, y=TRUE) -> (x = y?=w414:bool)
            n198 = Equal?(x=w418, y=w417) -> (x = y?=w413:bool)
            n199 = Equal?(x=w414, y=w413) -> (x = y?=w410:bool)
            n200 = control-ref of="Scan Line Time"() -> (w407:refnum<vi>)
            n201 = control-ref of="Scan Line Delay"() -> (w408:refnum<vi>)
            n202 = control-ref of="Scan Width"() -> (w409:refnum<vi>)
            n203 = case shown="True" w410 {
              tunnel: w411 -> [w419 w441]
              tunnel: [w419 w440] -> w406
              tunnel: w408 -> [_ w439]
              tunnel: w409 -> [_ w438]
              tunnel: w407 -> [_ w422]
              frame False {
              }
              frame True {
                n204 = property class="Camera"(reference=w441) -> (reference out=w440:refnum<k24>, "Settings"=w437:refnum<k24>)  [unwired: 1 in, 1 out]
                n205 = property class="CameraSettings"(reference=w437) -> (reference out=w427:refnum<k24>, error out=w433:errorcluster, "ScanLineDelay"=w436:refnum<k24>)  [unwired: 1 in]
                n206 = property class="PmNumericParam`1[[System.UInt32"(reference=w436, error in=w433) -> (reference out=w434:refnum<k24>, error out=w432:errorcluster, "Available"=w435:bool)
                n207 = case shown="True" w435 {
                  tunnel: w439 -> [_ w458]
                  tunnel: w434 -> [_ w457]
                  tunnel: w432 -> [w453 w456]
                  tunnel: [w453 w454] -> w428
                  frame False {
                  }
                  frame True {
                    n208 = property class="PmNumericParam`1[[System.UInt32"(reference=w457) -> (reference out=w461:refnum<k24>, "Max"=w459:u32, "Min"=w460:u32)  [unwired: 1 in, 1 out]
                    n209 = property class="DigNum (strict)"(reference=w458, error in=w456) -> (reference out=w465:refnum<vi>, error out=w455:errorcluster, "Value"=w464:dbl)
                    n210 = In Range and Coerce(upper limit=w459, x=w464, lower limit=w460) -> (coerced(x)=w463:dbl)  [unwired: 1 out]
                    n211 = property class="PmNumericParam`1[[System.UInt32"(reference=w461, "Current"=w463) -> (reference out=w462:refnum<k24>)  [unwired: 1 in, 1 out]
                    n212 = property class="PmNumericParam`1[[System.UInt32"(reference=w462) -> ("Current"=w466:u32)  [unwired: 1 in, 2 out]
                    n213 = property class="DigNum (strict)"(reference=w465, error in=w455, "Value"=w466) -> (error out=w454:errorcluster)  [unwired: 1 out]
                  }
                }
                n214 = property class="CameraSettings"(reference=w427) -> ("ScanWidth"=w426:refnum<k24>, "ScanLineTime"=w425:refnum<k24>)  [unwired: 1 in, 2 out]
                n215 = property class="PmNumericParam`1[[System.UInt32"(reference=w426, error in=w428) -> (reference out=w430:refnum<k24>, error out=w429:errorcluster, "Available"=w431:bool)
                n216 = case shown="True" w431 {
                  tunnel: w438 -> [_ w449]
                  tunnel: w430 -> [_ w452]
                  tunnel: w429 -> [w447 w450]
                  tunnel: [w447 w451] -> w421
                  frame False {
                  }
                  frame True {
                    n217 = property class="PmNumericParam`1[[System.UInt32"(reference=w452) -> ("Current"=w448:u32)  [unwired: 1 in, 2 out]
                    n218 = property class="DigNum (strict)"(reference=w449, error in=w450, "Value"=w448) -> (error out=w451:errorcluster)  [unwired: 1 out]
                  }
                }
                n219 = property class="PmNumericParam`1[[System.Int64,"(reference=w425, error in=w421) -> (reference out=w423:refnum<k24>, error out=w420:errorcluster, "Available"=w424:bool)
                n220 = case shown="True" w424 {
                  tunnel: w423 -> [_ w446]
                  tunnel: w422 -> [_ w444]
                  tunnel: w420 -> [_ w443]
                  frame False {
                  }
                  frame True {
                    n221 = property class="PmNumericParam`1[[System.Int64,"(reference=w446, error in=w443) -> (error out=w442:errorcluster, "Current"=w445:i64)  [unwired: 1 out]
                    n222 = property class="DigNum (strict)"(reference=w444, error in=w442, "Value"=w445) -> ()  [unwired: 2 out]
                  }
                }
              }
            }
          }
          event "Scan Width": Value Change {
            w478 = 0 items=["Idle", "Capturing"] ("Status")
            n223 = event-data() -> ()  [unwired: 1 in, 6 out]
            n224 = property class="Camera"(reference=w472) -> (reference out=w471:refnum<k24>, "IsOpen"=w477:bool, "Status"=w479:i32)  [unwired: 1 in, 1 out]
            n225 = Equal?(x=w477, y=TRUE) -> (x = y?=w475:bool)
            n226 = Equal?(x=w479, y=w478) -> (x = y?=w474:bool)
            n227 = Equal?(x=w475, y=w474) -> (x = y?=w473:bool)
            n228 = control-ref of="Scan Line Time"() -> (w467:refnum<vi>)
            n229 = control-ref of="Scan Width"() -> (w469:refnum<vi>)
            n230 = control-ref of="Scan Line Delay"() -> (w468:refnum<vi>)
            n231 = case shown="True" w473 {
              tunnel: w471 -> [w480 w502]
              tunnel: [w480 w501] -> w470
              tunnel: w469 -> [_ w500]
              tunnel: w468 -> [_ w499]
              tunnel: w467 -> [_ w484]
              frame False {
              }
              frame True {
                n232 = property class="Camera"(reference=w502) -> (reference out=w501:refnum<k24>, "Settings"=w498:refnum<k24>)  [unwired: 1 in, 1 out]
                n233 = property class="CameraSettings"(reference=w498) -> (reference out=w481:refnum<k24>, error out=w494:errorcluster, "ScanWidth"=w497:refnum<k24>)  [unwired: 1 in]
                n234 = property class="PmNumericParam`1[[System.UInt32"(reference=w497, error in=w494) -> (reference out=w495:refnum<k24>, error out=w493:errorcluster, "Available"=w496:bool)
                n235 = case shown="True" w496 {
                  tunnel: w500 -> [_ w519]
                  tunnel: w495 -> [_ w518]
                  tunnel: w493 -> [w514 w517]
                  tunnel: [w514 w515] -> w489
                  frame False {
                  }
                  frame True {
                    n236 = property class="PmNumericParam`1[[System.UInt32"(reference=w518) -> (reference out=w522:refnum<k24>, "Max"=w520:u32, "Min"=w521:u32)  [unwired: 1 in, 1 out]
                    n237 = property class="DigNum (strict)"(reference=w519, error in=w517) -> (reference out=w526:refnum<vi>, error out=w516:errorcluster, "Value"=w525:dbl)
                    n238 = In Range and Coerce(upper limit=w520, x=w525, lower limit=w521) -> (coerced(x)=w524:dbl)  [unwired: 1 out]
                    n239 = property class="PmNumericParam`1[[System.UInt32"(reference=w522, "Current"=w524) -> (reference out=w523:refnum<k24>)  [unwired: 1 in, 1 out]
                    n240 = property class="PmNumericParam`1[[System.UInt32"(reference=w523) -> ("Current"=w527:u32)  [unwired: 1 in, 2 out]
                    n241 = property class="DigNum (strict)"(reference=w526, error in=w516, "Value"=w527) -> (error out=w515:errorcluster)  [unwired: 1 out]
                  }
                }
                n242 = property class="CameraSettings"(reference=w481) -> ("ScanLineDelay"=w488:refnum<k24>, "ScanLineTime"=w487:refnum<k24>)  [unwired: 1 in, 2 out]
                n243 = property class="PmNumericParam`1[[System.UInt32"(reference=w488, error in=w489) -> (reference out=w491:refnum<k24>, error out=w490:errorcluster, "Available"=w492:bool)
                n244 = case shown="True" w492 {
                  tunnel: w499 -> [_ w510]
                  tunnel: w491 -> [_ w513]
                  tunnel: w490 -> [w508 w511]
                  tunnel: [w508 w512] -> w483
                  frame False {
                  }
                  frame True {
                    n245 = property class="PmNumericParam`1[[System.UInt32"(reference=w513) -> ("Current"=w509:u32)  [unwired: 1 in, 2 out]
                    n246 = property class="DigNum (strict)"(reference=w510, error in=w511, "Value"=w509) -> (error out=w512:errorcluster)  [unwired: 1 out]
                  }
                }
                n247 = property class="PmNumericParam`1[[System.Int64,"(reference=w487, error in=w483) -> (reference out=w485:refnum<k24>, error out=w482:errorcluster, "Available"=w486:bool)
                n248 = case shown="True" w486 {
                  tunnel: w485 -> [_ w507]
                  tunnel: w484 -> [_ w505]
                  tunnel: w482 -> [_ w504]
                  frame False {
                  }
                  frame True {
                    n249 = property class="PmNumericParam`1[[System.Int64,"(reference=w507, error in=w504) -> (error out=w503:errorcluster, "Current"=w506:i64)  [unwired: 1 out]
                    n250 = property class="DigNum (strict)"(reference=w505, error in=w503, "Value"=w506) -> ()  [unwired: 2 out]
                  }
                }
              }
            }
          }
          event "Trigger In Behaviour", "Trigger Out Behaviour": Value Change {
            n251 = event-data() -> ()  [unwired: 1 in, 6 out]
            n252 = local read "Camera Status"() -> (w528:bool)
            n253 = case shown="True" w528 {
              tunnel: w531 -> [w533 w537]
              tunnel: [w533 w534] -> w530
              frame False {
                n254 = One Button Dialog(message="Camera is not open") -> ()  [unwired: 1 in, 1 out]
              }
              frame True {
                w542 = 0 items=["Idle", "Capturing"] ("Status")
                n255 = property class="Camera"(reference=w537) -> (reference out=w535:refnum<k24>, "IsOpen"=w541:bool, "Status"=w543:i32)  [unwired: 1 in, 1 out]
                n256 = Equal?(x=w541, y=TRUE) -> (x = y?=w539:bool)
                n257 = Equal?(x=w543, y=w542) -> (x = y?=w538:bool)
                n258 = Equal?(x=w539, y=w538) -> (x = y?=w536:bool)
                n259 = case shown="True" w536 {
                  tunnel: w535 -> [w544 w566]
                  tunnel: [w544 w558] -> w534
                  frame False {
                  }
                  frame True {
                    n260 = property class="Camera"(reference=w566) -> (reference out=w558:refnum<k24>, "Settings"=w553:refnum<k24>)  [unwired: 1 in, 1 out]
                    n261 = control-ref of="Trigger In Behaviour"() -> (w548:refnum<vi>)
                    n262 = control-ref of="Trigger Mode"() -> (w549:refnum<vi>)
                    n263 = control-ref of="Trigger Out Behaviour"() -> (w554:refnum<vi>)
                    n264 = control-ref of="Exp. out"() -> (w555:refnum<vi>)
                    n265 = property class="CameraSettings"(reference=w553) -> (reference out=w552:refnum<k24>, "ExposureTime"=w551:refnum<k24>, "ExposureMode"=w545:refnum<k24>, "ExposeOutMode"=w550:refnum<k24>)  [unwired: 1 in, 1 out]
                    n266 = property class="PmEnumParam"(reference=w550) -> (reference out=w556:refnum<k24>, "Available"=w557:bool)  [unwired: 1 in, 1 out]
                    n267 = property class="PmEnumParam"(reference=w545) -> (reference out=w547:refnum<k24>, "Available"=w546:bool)  [unwired: 1 in, 1 out]
                    n268 = property class="PmNumericParam`1[[System.UInt64"(reference=w551) -> (reference out=w563:refnum<k24>, "Max"=w565:u64, "Min"=w564:u64)  [unwired: 1 in, 1 out]
                    n269 = case shown="True" w557 {
                      tunnel: w556 -> [_ w591]
                      tunnel: w555 -> [_ w585]
                      tunnel: w554 -> [_ w582]
                      frame False {
                      }
                      frame True {
                        n270 = property class="CmbBox"(reference=w582) -> (reference out=w584:refnum<vi>, "Strings[]"=w592:string[])  [unwired: 1 in, 1 out]
                        n271 = property class="CmbBox"(reference=w584) -> ("Value"=w583:string)  [unwired: 1 in, 2 out]
                        n272 = while {
                          tunnel: w592 -> [w596] mode=indexing
                          tunnel: [w594] -> w589
                          tunnel: w583 -> [w593]
                          i -> [w594]
                          stop <- w595 stop-if-true
                          n273 = Equal?(x=w596, y=w593) -> (x = y?=w595:bool)
                        }
                        n274 = property class="PmEnumParam"(reference=w591) -> (reference out=w588:refnum<k24>, "Options"=w590:refnum<k24>)  [unwired: 1 in, 1 out]
                        n275 = invoke class="PmReadOnlyObservableCollection`" method="get_Item"(reference=w590, "index"=w589) -> ("get_Item"=w587:refnum<k24>)  [unwired: 2 in, 3 out]
                        n276 = property class="PmEnumItem"(reference=w587) -> ("Value"=w586:i32)  [unwired: 1 in, 2 out]
                        n277 = property class="PmEnumParam"(reference=w588, "Current"=w587) -> ()  [unwired: 1 in, 2 out]
                        n278 = property class="DigNum (strict)"(reference=w585, "Value"=w586) -> ()  [unwired: 1 in, 2 out]
                      }
                    }
                    n279 = case shown="True" w546 {
                      tunnel: w547 -> [_ w576]
                      tunnel: w549 -> [_ w570]
                      tunnel: w548 -> [_ w567]
                      frame False {
                      }
                      frame True {
                        n280 = property class="CmbBox"(reference=w567) -> (reference out=w569:refnum<vi>, "Strings[]"=w577:string[])  [unwired: 1 in, 1 out]
                        n281 = property class="CmbBox"(reference=w569) -> ("Value"=w568:string)  [unwired: 1 in, 2 out]
                        n282 = while {
                          tunnel: w577 -> [w581] mode=indexing
                          tunnel: [w579] -> w574
                          tunnel: w568 -> [w578]
                          i -> [w579]
                          stop <- w580 stop-if-true
                          n283 = Equal?(x=w581, y=w578) -> (x = y?=w580:bool)
                        }
                        n284 = property class="PmEnumParam"(reference=w576) -> (reference out=w573:refnum<k24>, "Options"=w575:refnum<k24>)  [unwired: 1 in, 1 out]
                        n285 = invoke class="PmReadOnlyObservableCollection`" method="get_Item"(reference=w575, "index"=w574) -> ("get_Item"=w572:refnum<k24>)  [unwired: 2 in, 3 out]
                        n286 = property class="PmEnumItem"(reference=w572) -> ("Value"=w571:i32)  [unwired: 1 in, 2 out]
                        n287 = property class="PmEnumParam"(reference=w573, "Current"=w572) -> ()  [unwired: 1 in, 2 out]
                        n288 = property class="DigNum (strict)"(reference=w570, "Value"=w571) -> ()  [unwired: 1 in, 2 out]
                      }
                    }
                    n289 = local read "Exposure Time"() -> (w560:dbl)
                    n290 = In Range and Coerce(upper limit=w565, x=w560, lower limit=w564) -> (coerced(x)=w561:dbl)  [unwired: 1 out]
                    n291 = property class="CameraSettings"(reference=w552, "Exposure"=w561) -> ()  [unwired: 1 in, 2 out]
                    n292 = property class="PmNumericParam`1[[System.UInt64"(reference=w563, "Current"=w561) -> (reference out=w562:refnum<k24>)  [unwired: 1 in, 1 out]
                    n293 = property class="PmNumericParam`1[[System.UInt64"(reference=w562) -> ("Current"=w559:u64)  [unwired: 1 in, 2 out]
                    n294 = local write "Exposure Time"(w559) -> ()
                  }
                }
              }
            }
          }
          event "Get ROI": Value Change {
            n295 = event-data() -> ()  [unwired: 1 in, 6 out]
            n296 = case shown="True" "Get ROI" {
              tunnel: w598 -> [w600 w603]
              tunnel: [w600 w602] -> w597
              frame False {
              }
              frame True {
                n297 = local read "Camera Status"() -> (w601:bool)
                n298 = case shown="True" w601 {
                  tunnel: w603 -> [w605 w609]
                  tunnel: [w605 w606] -> w602
                  frame False {
                    n299 = One Button Dialog(message="Camera is not open") -> ()  [unwired: 1 in, 1 out]
                  }
                  frame True {
                    w614 = 0 items=["Idle", "Capturing"] ("Status")
                    n300 = property class="Camera"(reference=w609) -> (reference out=w608:refnum<k24>, "IsOpen"=w613:bool, "Status"=w615:i32)  [unwired: 1 in, 1 out]
                    n301 = Equal?(x=w613, y=TRUE) -> (x = y?=w611:bool)
                    n302 = Equal?(x=w615, y=w614) -> (x = y?=w610:bool)
                    n303 = Equal?(x=w611, y=w610) -> (x = y?=w607:bool)
                    n304 = case shown="True" w607 {
                      tunnel: w608 -> [w617 w625]
                      tunnel: [w617 w624] -> w606
                      frame False {
                        n305 = One Button Dialog(message="Camera must be idle.") -> ()  [unwired: 1 in, 1 out]
                      }
                      frame True {
                        n306 = property class="Camera"(reference=w625) -> (reference out=w624:refnum<k24>, "Settings"=w623:refnum<k24>)  [unwired: 1 in, 1 out]
                        n307 = property class="CameraSettings"(reference=w623) -> ("Regions"=w622:refnum<k24>)  [unwired: 1 in, 2 out]
                        n308 = property class="PmObservableCollection`1[[PVCam"(reference=w622) -> (reference out=w618:refnum<k24>, "Count"=w621:i32)  [unwired: 1 in, 1 out]
                        n309 = Greater?(x=w621, y=0) -> (0:w619:bool)
                        n310 = case shown="True" w619 {
                          tunnel: w618 -> [_ w627]
                          frame False {
                            n311 = One Button Dialog(message="ROI is not created.") -> ()  [unwired: 1 in, 1 out]
                          }
                          frame True {
                            n312 = invoke class="PmObservableCollection`1[[PVCam" method="get_Item"(reference=w627, "index"=0) -> ("get_Item"=w633:refnum<k24>)  [unwired: 2 in, 3 out]
                            n313 = property class="PmRegion"(reference=w633) -> ("Height"=w631:u16, "Width"=w630:u16, "X"=w629:u16, "Y"=w628:u16)  [unwired: 1 in, 2 out]
                            n314 = local write "Height"(w631) -> ()
                            n315 = local write "Width"(w630) -> ()
                            n316 = local write "X"(w629) -> ()
                            n317 = local write "Y"(w628) -> ()
                          }
                        }
                      }
                    }
                  }
                }
              }
            }
          }
          event "X", "Width", "Y", "Height": Value Change {
            n318 = event-data() -> ()  [unwired: 1 in, 6 out]
            n319 = local read "Camera Status"() -> (w636:bool)
            n320 = case shown="True" w636 {
              tunnel: w635 -> [w637 w640]
              tunnel: [w637 w638] -> w634
              frame False {
              }
              frame True {
                w646 = 0 items=["Idle", "Capturing"] ("Status")
                n321 = property class="Camera"(reference=w640) -> (reference out=w639:refnum<k24>, "IsOpen"=w645:bool, "Status"=w647:i32)  [unwired: 1 in, 1 out]
                n322 = Equal?(x=w645, y=TRUE) -> (x = y?=w643:bool)
                n323 = Equal?(x=w647, y=w646) -> (x = y?=w642:bool)
                n324 = Equal?(x=w643, y=w642) -> (x = y?=w641:bool)
                n325 = case shown="True" w641 {
                  tunnel: w639 -> [w648 w650]
                  tunnel: [w648 w649] -> w638
                  frame False {
                  }
                  frame True {
                    n326 = flat-sequence {
                      tunnel: w650 -> [w698]
                      tunnel: [w697] -> w649
                      frame #0 {
                        # "if (!( x >= 0\n            && (x+width) <= full_width\n            &&  0 < width \n            && y >= 0\n            && (y+height) <= full_height\n            && 0 < height ))\n        {\n           printf(\"Incorrect range for a ROI. \\n\");\n        }"
                        n327 = local read "Width"() -> (w666:u16)
                        n328 = local read "Height"() -> (w664:u16)
                        n329 = local read "Full CCD Height"() -> (w660:u16)
                        n330 = local read "Full CCD Width"() -> (w662:u16)
                        n331 = local read "X"() -> (w667:u16)
                        n332 = local read "Y"() -> (w663:u16)
                        n333 = local read "Height"() -> (w655:u16)
                        n334 = Add(x=w667, y=w666) -> (x+y=w661:u16)
                        n335 = local read "Width"() -> (w658:u16)
                        n336 = Add(x=w664, y=w663) -> (x+y=w659:u16)
                        n337 = local read "X"() -> (w668:u16)
                        n338 = local read "Y"() -> (w665:u16)
                        n339 = Less Or Equal?(x=w659, y=w660) -> (x <= y?=w675:bool)
                        n340 = Less Or Equal?(x=w661, y=w662) -> (x <= y?=w678:bool)
                        n341 = Less?(x=u16 0 ("y"), y=w655) -> (x < y?=w674:bool)
                        n342 = Greater Or Equal?(x=w668, y=u16 0) -> (x >= y?=w679:bool)
                        n343 = Less?(x=u16 0 ("y"), y=w658) -> (x < y?=w677:bool)
                        n344 = Greater Or Equal?(x=w665, y=u16 0) -> (x >= y?=w676:bool)
                        n345 = And(x=w675, y=w674) -> (x .and. y?=w670:bool)
                        n346 = And(x=w679, y=w678) -> (x .and. y?=w673:bool)
                        n347 = And(x=w677, y=w676) -> (x .and. y?=w672:bool)
                        n348 = And(x=w673, y=w672) -> (x .and. y?=w671:bool)
                        n349 = And(x=w671, y=w670) -> (x .and. y?=w669:bool)
                        n350 = case shown="False" w669 {
                          tunnel: [w683 w690] -> w654
                          tunnel: [u16 0 ("X") w689] -> w651
                          tunnel: [u16 0 ("Y") w688] -> w652
                          tunnel: [w684 w687] -> w653
                          frame False {
                            n351 = local read "Full CCD Height"() -> (w684:u16)
                            n352 = local read "Full CCD Width"() -> (w683:u16)
                            n353 = One Button Dialog(message="Wrong ROI ! Resetting to full CCD") -> ()  [unwired: 1 in, 1 out]
                          }
                          frame True {
                            n354 = local read "Height"() -> (w687:u16)
                            n355 = local read "Width"() -> (w690:u16)
                            n356 = local read "X"() -> (w689:u16)
                            n357 = local read "Y"() -> (w688:u16)
                          }
                        }
                        n358 = local write "Width"(w654) -> ()
                        n359 = local write "X"(w651) -> ()
                        n360 = local write "Y"(w652) -> ()
                        n361 = local write "Height"(w653) -> ()
                      }
                      frame #1 {
                        n362 = property class="Camera"(reference=w698) -> (reference out=w697:refnum<k24>, "Settings"=w696:refnum<k24>)  [unwired: 1 in, 1 out]
                        n363 = property class="CameraSettings"(reference=w696) -> ("Regions"=w695:refnum<k24>)  [unwired: 1 in, 2 out]
                        n364 = property class="PmObservableCollection`1[[PVCam"(reference=w695) -> (reference out=w691:refnum<k24>, "Count"=w694:i32)  [unwired: 1 in, 1 out]
                        n365 = Greater?(x=w694, y=0) -> (0:w692:bool)
                        n366 = case shown="True" w692 {
                          tunnel: w691 -> [_ w704]
                          frame False {
                            n367 = One Button Dialog(message="ROI is not created.") -> ()  [unwired: 1 in, 1 out]
                          }
                          frame True {
                            n368 = invoke class="PmObservableCollection`1[[PVCam" method="get_Item"(reference=w704, "index"=0) -> ("get_Item"=w706:refnum<k24>)  [unwired: 2 in, 3 out]
                            n369 = local read "Height"() -> (w703:u16)
                            n370 = local read "Width"() -> (w702:u16)
                            n371 = local read "X"() -> (w701:u16)
                            n372 = local read "Y"() -> (w700:u16)
                            n373 = property class="PmRegion"(reference=w706, "Height"=w703, "Width"=w702, "X"=w701, "Y"=w700) -> ()  [unwired: 1 in, 2 out]
                          }
                        }
                      }
                    }
                  }
                }
              }
            }
          }
          event "Path", "FramesToCapture": Value Change {
            n374 = event-data() -> ()  [unwired: 1 in, 6 out]
            n375 = local read "Camera Status"() -> (w709:bool)
            n376 = case shown="True" w709 {
              tunnel: w708 -> [w710 w713]
              tunnel: [w710 w711] -> w707
              frame False {
              }
              frame True {
                w719 = 0 items=["Idle", "Capturing"] ("Status")
                n377 = property class="Camera"(reference=w713) -> (reference out=w712:refnum<k24>, "IsOpen"=w718:bool, "Status"=w720:i32)  [unwired: 1 in, 1 out]
                n378 = Equal?(x=w718, y=TRUE) -> (x = y?=w716:bool)
                n379 = Equal?(x=w720, y=w719) -> (x = y?=w715:bool)
                n380 = Equal?(x=w716, y=w715) -> (x = y?=w714:bool)
                n381 = case shown="True" w714 {
                  tunnel: w712 -> [w721 w724]
                  tunnel: [w721 w723] -> w711
                  frame False {
                  }
                  frame True {
                    n382 = property class="Camera"(reference=w724) -> (reference out=w723:refnum<k24>, "Settings"=w727:refnum<k24>, "AcquisitionBuffer"=w728:refnum<k24>)  [unwired: 1 in, 1 out]
                    n383 = Path To String(path="Path") -> (string=w731:string)
                    n384 = Concatenate Strings(w731, "\\" ("string")) -> (w733:string)
                    "SavingPath" <- w733
                    n385 = property class="AcqBuffer"(reference=w728, "BufferSize"="FramesToCapture", "ImageSavingPath"=w733, "BigTiffRequired"=FALSE) -> (reference out=w729:refnum<k24>)  [unwired: 1 in, 1 out]
                    n386 = property class="CameraSettings"(reference=w727, "FramesToCapture"="FramesToCapture") -> ()  [unwired: 1 in, 2 out]
                    n387 = property class="AcqBuffer"(reference=w729) -> ("ImageSavingPath"=w730:string)  [unwired: 1 in, 2 out]
                    n388 = local write "SavingPath"(w730) -> ()
                  }
                }
              }
            }
          }
          event "Full CCD": Value Change {
            n389 = event-data() -> ()  [unwired: 1 in, 6 out]
            n390 = case shown="True" "Full CCD" {
              tunnel: w735 -> [w737 w740]
              tunnel: [w737 w739] -> w734
              frame False {
              }
              frame True {
                n391 = local read "Camera Status"() -> (w738:bool)
                n392 = case shown="True" w738 {
                  tunnel: w740 -> [w742 w746]
                  tunnel: [w742 w743] -> w739
                  frame False {
                    n393 = One Button Dialog(message="Camera is not open") -> ()  [unwired: 1 in, 1 out]
                  }
                  frame True {
                    w751 = 0 items=["Idle", "Capturing"] ("Status")
                    n394 = property class="Camera"(reference=w746) -> (reference out=w745:refnum<k24>, "IsOpen"=w750:bool, "Status"=w752:i32)  [unwired: 1 in, 1 out]
                    n395 = Equal?(x=w750, y=TRUE) -> (x = y?=w748:bool)
                    n396 = Equal?(x=w752, y=w751) -> (x = y?=w747:bool)
                    n397 = Equal?(x=w748, y=w747) -> (x = y?=w744:bool)
                    n398 = case shown="True" w744 {
                      tunnel: w745 -> [w753 w762]
                      tunnel: [w753 w761] -> w743
                      frame False {
                      }
                      frame True {
                        n399 = property class="Camera"(reference=w762) -> (reference out=w761:refnum<k24>, "Settings"=w760:refnum<k24>)  [unwired: 1 in, 1 out]
                        n400 = property class="CameraSettings"(reference=w760) -> (reference out=w754:refnum<k24>, "Regions"=w755:refnum<k24>)  [unwired: 1 in, 1 out]
                        n401 = property class="PmObservableCollection`1[[PVCam"(reference=w755) -> (reference out=w756:refnum<k24>, "Count"=w759:i32)  [unwired: 1 in, 1 out]
                        n402 = Greater?(x=w759, y=0) -> (0:w757:bool)
                        n403 = case shown="True" w757 {
                          tunnel: w756 -> [_ _]
                          tunnel: w755 -> [_ w771]
                          tunnel: w754 -> [_ w765]
                          frame False {
                          }
                          frame True {
                            n404 = invoke class="PmObservableCollection`1[[PVCam" method="RemoveAt"(reference=w771, "index"=0) -> ()  [unwired: 2 in, 4 out]
                            n405 = property class="CameraSettings"(reference=w765) -> ("SensorWidth"=w767:refnum<k24>)  [unwired: 1 in, 2 out]
                            n406 = property class="CameraSettings"(reference=w765) -> ("SensorHeight"=w768:refnum<k24>)  [unwired: 1 in, 2 out]
                            n407 = property class="PmNumericParam`1[[System.UInt32"(reference=w767) -> ("Current"=w766:u32)  [unwired: 1 in, 2 out]
                            n408 = property class="PmNumericParam`1[[System.UInt32"(reference=w768) -> ("Current"=w769:u32)  [unwired: 1 in, 2 out]
                            n409 = local write "Y"(0 ("index")) -> ()
                            n410 = local write "Width"(w766) -> ()
                            n411 = local write "Height"(w769) -> ()
                            n412 = local write "X"(0 ("index")) -> ()
                          }
                        }
                      }
                    }
                  }
                }
              }
            }
          }
          event "Live start": Value Change {
            n413 = event-data() -> ()  [unwired: 1 in, 6 out]
            n414 = case shown="True" "Live start" {
              tunnel: w774 -> [w776 w779]
              tunnel: [w776 w778] -> w773
              frame False {
              }
              frame True {
                n415 = local read "Camera Status"() -> (w777:bool)
                n416 = case shown="True" w777 {
                  tunnel: w779 -> [w780 w785]
                  tunnel: [w780 w783] -> w778
                  frame False {
                    n417 = One Button Dialog(message="Camera is not open") -> ()  [unwired: 1 in, 1 out]
                  }
                  frame True {
                    w790 = 0 items=["Idle", "Capturing"] ("Status")
                    n418 = property class="Camera"(reference=w785) -> (reference out=w784:refnum<k24>, "IsOpen"=w789:bool, "Status"=w791:i32)  [unwired: 1 in, 1 out]
                    n419 = Equal?(x=w789, y=TRUE) -> (x = y?=w787:bool)
                    n420 = Equal?(x=w791, y=w790) -> (x = y?=w786:bool)
                    n421 = Equal?(x=w787, y=w786) -> (x = y?=w782:bool)
                    n422 = case shown="True" w782 {
                      tunnel: w784 -> [w793 w795]
                      tunnel: [w793 w796] -> w783
                      frame False {
                        n423 = local write "Live"(FALSE ("Live 2")) -> ()
                      }
                      frame True {
                        n424 = flat-sequence {
                          tunnel: w795 -> [w801]
                          tunnel: [w798] -> w794
                          frame #0 {
                            n425 = property class="Camera"(reference=w801) -> (reference out=w798:refnum<k24>, "AcquisitionBuffer"=w800:refnum<k24>)  [unwired: 1 in, 1 out]
                            n426 = property class="AcqBuffer"(reference=w800, "BufferSize"=100) -> ()  [unwired: 1 in, 2 out]
                          }
                        }
                        n427 = local write "Live"(TRUE ("Live")) -> ()
                        n428 = invoke class="Camera" method="StartLive"(reference=w794) -> (reference out=w796:refnum<k24>)  [unwired: 2 in, 2 out]
                      }
                    }
                  }
                }
              }
            }
          }
          event "Live stop": Value Change {
            n429 = event-data() -> ()  [unwired: 1 in, 6 out]
            n430 = case shown="True" "Live stop" {
              tunnel: w803 -> [w805 w808]
              tunnel: [w805 w807] -> w802
              frame False {
              }
              frame True {
                n431 = local read "Camera Status"() -> (w806:bool)
                n432 = case shown="False" w806 {
                  tunnel: w808 -> [w810 w820]
                  tunnel: [w810 w817] -> w807
                  frame False {
                    n433 = One Button Dialog(message="Camera is not open") -> ()  [unwired: 1 in, 1 out]
                  }
                  frame True {
                    w815 = 1 items=["Idle", "Capturing"] ("Status")
                    n434 = property class="Camera"(reference=w820) -> (reference out=w818:refnum<k24>, "IsOpen"=w814:bool, "Status"=w816:i32)  [unwired: 1 in, 1 out]
                    n435 = Equal?(x=w816, y=w815) -> (x = y?=w811:bool)
                    n436 = Equal?(x=w814, y=TRUE) -> (x = y?=w812:bool)
                    n437 = Equal?(x=w812, y=w811) -> (x = y?=w819:bool)
                    n438 = case shown="True" w819 {
                      tunnel: w818 -> [w821 w824]
                      tunnel: [w821 w823] -> w817
                      frame False {
                      }
                      frame True {
                        n439 = invoke class="Camera" method="Stop"(reference=w824) -> (reference out=w823:refnum<k24>)  [unwired: 2 in, 2 out]
                        n440 = local write "Live"(FALSE ("Live 2")) -> ()
                      }
                    }
                  }
                }
              }
            }
          }
          event "Uninit": Value Change {
            n441 = event-data() -> ()  [unwired: 1 in, 6 out]
            n442 = case shown="True" "Uninit" {
              tunnel: w829 -> [w831 w835]
              tunnel: [w831 w834] -> w828
              tunnel: [FALSE ("Camera Status") w832] -> w826
              frame False {
              }
              frame True {
                n443 = local read "Camera Status"() -> (w833:bool)
                n444 = case shown="True" w833 {
                  tunnel: w835 -> [w837 w842]
                  tunnel: [w837 w841] -> w834
                  tunnel: [FALSE ("Camera Status") w840] -> w832
                  frame False {
                  }
                  frame True {
                    n445 = local read "Live"() -> (w838:bool)
                    n446 = Not(x=w838) -> (.not. x?=w839:bool)
                    n447 = case shown="True" w839 {
                      tunnel: w842 -> [w844 w847]
                      tunnel: [w844 w846] -> w841
                      tunnel: [FALSE ("Camera Status") w845] -> w840
                      frame False {
                      }
                      frame True {
                        n448 = flat-sequence {
                          tunnel: w847 -> [w850]
                          tunnel: [w849] -> w848
                          tunnel: [w853] -> w846
                          tunnel: w848 -> [w853]
                          tunnel: [TRUE ("Camera Status")] -> w845
                          frame #0 {
                            n449 = invoke class="Camera" method="Close"(reference=w850) -> (reference out=w849:refnum<k24>)  [unwired: 2 in, 2 out]
                          }
                          frame #1 {
                            n450 = local write "Camera Status"(FALSE ("Camera Status")) -> ()
                          }
                        }
                      }
                    }
                  }
                }
              }
            }
          }
        }
      }
    }
    frame #2 {
      n451 = invoke class="Library" method="Release"(reference=w855) -> (reference out=w856:refnum<k24>)  [unwired: 2 in, 2 out]
      n452 = Wait (ms)(milliseconds to wait=u32 100) -> ()  [unwired: 1 out]
      n453 = Close Reference(reference=w856) -> ()  [unwired: 1 in, 1 out]
    }
    frame #3 {
      n454 = invoke class="GC" method="Collect"() -> ()  [unwired: 3 in, 3 out]
    }
  }
  n455 = control-ref of="Exp. out"() -> (w8:refnum<vi>)
  n456 = property class="DigNum (strict)"(reference=w8, "Visible"=FALSE) -> ()  [unwired: 1 in, 2 out]
  n457 = control-ref of="Trigger Mode"() -> (w7:refnum<vi>)
  n458 = property class="DigNum (strict)"(reference=w7, "Visible"=FALSE) -> ()  [unwired: 1 in, 2 out]
  n459 = control-ref of="Trigger Out Behaviour"() -> (w13:refnum<vi>)
  n460 = control-ref of="Exp. out"() -> (w11:refnum<vi>)
  n461 = property class="DigNum (strict)"(reference=w11, "Value"=0) -> ()  [unwired: 1 in, 2 out]
  n462 = property class="CmbBox"(reference=w13, "Value"="") -> ()  [unwired: 1 in, 2 out]
  n463 = local write "Camera Status"(FALSE ("Camera Status")) -> ()
  n464 = property on="Scan Width" class="DigNum (strict)"("DisabledEnum"=w16) -> ()  [unwired: 2 in, 2 out]
  n465 = property on="Scan Line Delay" class="DigNum (strict)"("DisabledEnum"=w16) -> ()  [unwired: 2 in, 2 out]
  n466 = control-ref of="Scan Line Delay"() -> (w19:refnum<vi>)
  n467 = control-ref of="Scan Width"() -> (w22:refnum<vi>)
  n468 = control-ref of="Scan Line Time"() -> (w18:refnum<vi>)
  n469 = control-ref of="Scan Direction"() -> (w25:refnum<vi>)
  n470 = control-ref of="Scan Mode"() -> (w28:refnum<vi>)
  n471 = property class="CmbBox"(reference=w28, "Value"="", "Strings[]"=string[] [] ("Strings []")) -> ()  [unwired: 1 in, 2 out]
  n472 = property class="DigNum (strict)"(reference=w19, "Value"=0.0) -> ()  [unwired: 1 in, 2 out]
  n473 = property class="CmbBox"(reference=w25, "Strings[]"=string[] [] ("Strings []"), "Value"="") -> ()  [unwired: 1 in, 2 out]
  n474 = property class="DigNum (strict)"(reference=w22, "Value"=0.0) -> ()  [unwired: 1 in, 2 out]
  n475 = property class="DigNum (strict)"(reference=w18, "Value"=0.0) -> ()  [unwired: 1 in, 2 out]
  n476 = local write "Scan Direction Reset"(FALSE ("Boolean")) -> ()
  n477 = control-ref of="FramesToCapture"() -> (w5:refnum<vi>)
  n478 = control-ref of="Path"() -> (w3:refnum<vi>)
  n479 = String To Path(string="C:\\Users\\lightsheetscope\\Desktop") -> (path=w1:path)
  n480 = property class="DigNum (strict)"(reference=w5, "Value"=10) -> ()  [unwired: 1 in, 2 out]
  n481 = property class="Path"(reference=w3, "Value"=w1) -> ()  [unwired: 1 in, 2 out]
  "Boolean" <- FALSE ("Boolean")
